vi "Main v0.01.vi"() -> ()   [LabVIEW 2017]
doc: "This vi is the main vi for startup. It has the following loops:\n\n1. The Event Handling Loop generates messages based on user interface actions.\n\n2. The Message Handling Loop processes messages generated by the Event Handling Loop, or by other messages. The messages are string values, so new messages can be added easily to the Message Cases case structure in the Message Handling Loop. Each message cluster can also provide an optional value for Message Data, which is a variant that can be converted to whatever message-specific data is required.\n\n3. The Auto Loop runs the endurance tests\n\n4. The Towerlight loop maintains the status of the towerlight based on machine running\n\n--------------------\n\nv1.7:\n- Added Sense ON Delay to the Tolerances Cluster making it user editable\n- Config file for writing tolerances is now changed to config.ini inside data folder\n\nv1.6:\n- Added a error dialog before starting loops to display errors\n- Backup nce file creation\n- UAC logger Updated\n\nv1.51:\n- Updated UAC\n\nChangelog\nv1.43:\n- Fixed bug for display of updated motor calibrration data (read new value from queue)\n- Fixed bug for speed calibration\n\nv1.41:\n- Added debouncing of E-Stop (Autoloop)\n- Modified timeout error algorithm (Procedure Run)\n- Text description on Settings screen\n\nv1.4:\n- Don;t allow to Run the test until correct procedure is selected\n\nv1.3:\n- UI updated for Calibration Screen\n\nv1.2:\n- UI Improvement:\n - Settings mode style updated\n\nv1.12:\n- Manual mode updated for ECU\n- Maintenance mode E-Stop colour changed\n\nv1.11:\n- Made towerlight handling into subVI\n\nv1.1:\n- Climate Chamber error convert to warning\n- View procedure puts same value into its indicators for next run. This basically means current procedure of the motor will show even if you do not change to another motor and return.\n- Added View Log feature\n- Added View Details feature\n\nv1.0:\n- Climate chamber integration completion\n- Maintenance mode along with climate UI\n- UI changes to auto screen\n\nv0.91:\n- Towerlight Buzzer intermittently\n- Remarks indicator added to Auto Mode\n\nv0.8:\n- Pause, Start, Stop, Procedure View updated\n- Diection indicator added\n- Motor Select enable/disable added\n\nv0.7:\n- Indicators & graphs updated for auto mode"
uses:
  support/Message Queue/Message Queue.lvlib
  <vilib>/Utility/error.llb/Error Cluster From Error Code.vi
  support/User Event - Stop/User Event - Stop.lvlib
  support/Message Queue/Enqueue Message (Single).vi
  <vilib>/ErrorRing/Error Ring.xnode
  support/GV/Towerlight GV.vi
  controls/Towerlight.ctl
  controls/FGV DO.ctl
  <resource>/objmgr/daqmx.rc
  controls/Auto States v0.2.ctl
  controls/AC Results.ctl
  controls/Update Measurements.ctl
  controls/Specifications.ctl
  controls/All Specs.ctl
  controls/Main Tabs.ctl
  controls/FGV AO.ctl
  GV/All Inputs.vi
  GV/Specs.vi
  controls/Model Name.ctl
  controls/Auto.ctl
  controls/SACB DI.ctl
panel:
  in  "Number":string="ID" caption="No"
  in  "Shift":string="ID"
  in  "BSL":bool
  out "Numeric Control":i32
  out "Array":string[](array[string])
  out "Total Time":dbl caption="Total Time (s)"
  in  "output cluster":T1={"LH"={"Go Up"={"Min Speed"=10.0, "Max Speed"=250.0, "Min Time"=0.5, "Max Time"=5.3, "Min Run Current"=0.0, "Max Run Current"=10.0, "Min Stall Current"=0.0, "Max Stall Current"=25.0, "Min Stall Force"=170.0, "Max Stall Force"=320.0, "Min Stroke"=170.0, "Max Stroke"=350.0}, "Go Down"={"Min Speed"=10.0, "Max Speed"=250.0, "Min Travel Time"=0.5, "Max Travel Time"=5.3, "Min Run Current"=0.0, "Max Run Current"=10.0}, "Shipping"={"Min Distance"=0.0, "Max Distance"=25.0, "Setpoint"=5.0}, "Anti-Pinch"={"Min Force"=5.0, "Max Force"=15.0}}, "RH"={"Go Up"={"Min Speed"=10.0, "Max Speed"=250.0, "Min Time"=0.5, "Max Time"=4.3, "Min Run Current"=0.0, "Max Run Current"=10.0, "Min Stall Current"=0.0, "Max Stall Current"=25.0, "Min Stall Force"=170.0, "Max Stall Force"=320.0, "Min Stroke"=170.0, "Max Stroke"=350.0}, "Go Down"={"Min Speed"=10.0, "Max Speed"=250.0, "Min Travel Time"=0.5, "Max Travel Time"=5.3, "Min Run Current"=0.0, "Max Run Current"=10.0}, "Shipping"={"Min Distance"=0.0, "Max Distance"=25.0, "Setpoint"=5.0}, "Anti-Pinch"={"Min Force"=5.0, "Max Force"=15.0}}, "W 601 FR RH Std"={"Go Up"={"Min Speed"=10.0, "Max Speed"=250.0, "Min Time"=0.5, "Max Time"=4.3, "Min Run Current"=0.0, "Max Run Current"=10.0, "Min Stall Current"=0.0, "Max Stall Current"=25.0, "Min Stall Force"=170.0, "Max Stall Force"=320.0, "Min Stroke"=254.4, "Max Stroke"=270.4}, "Go Down"={"Min Speed"=10.0, "Max Speed"=250.0, "Min Travel Time"=0.5, "Max Travel Time"=4.3, "Min Run Current"=0.0, "Max Run Current"=10.0}, "Shipping"={"Min Distance"=5.0, "Max Distance"=15.0, "Setpoint"=5.0}, "Anti-Pinch"={"Min Force"=5.0, "Max Force"=15.0}}, "W 601 FR LH Std"={"Go Up"={"Min Speed"=10.0, "Max Speed"=250.0, "Min Time"=0.5, "Max Time"=4.3, "Min Run Current"=0.0, "Max Run Current"=10.0, "Min Stall Current"=0.0, "Max Stall Current"=25.0, "Min Stall Force"=170.0, "Max Stall Force"=320.0, "Min Stroke"=254.4, "Max Stroke"=270.4}, "Go Down"={"Min Speed"=10.0, "Max Speed"=250.0, "Min Travel Time"=0.5, "Max Travel Time"=4.3, "Min Run Current"=0.0, "Max Run Current"=10.0}, "Shipping"={"Min Distance"=5.0, "Max Distance"=15.0, "Setpoint"=5.0}, "Anti-Pinch"={"Min Force"=5.0, "Max Force"=15.0}}, "W 601 RR RH Std"={"Go Up"={"Min Speed"=10.0, "Max Speed"=250.0, "Min Time"=0.5, "Max Time"=4.3, "Min Run Current"=0.0, "Max Run Current"=10.0, "Min Stall Current"=0.0, "Max Stall Current"=25.0, "Min Stall Force"=170.0, "Max Stall Force"=320.0, "Min Stroke"=254.4, "Max Stroke"=270.4}, "Go Down"={"Min Speed"=10.0, "Max Speed"=250.0, "Min Travel Time"=0.5, "Max Travel Time"=4.3, "Min Run Current"=0.0, "Max Run Current"=10.0}, "Shipping"={"Min Distance"=5.0, "Max Distance"=15.0, "Setpoint"=5.0}, "Anti-Pinch"={"Min Force"=5.0, "Max Force"=15.0}}, "W 601 RR LH Std"={"Go Up"={"Min Speed"=10.0, "Max Speed"=250.0, "Min Time"=0.5, "Max Time"=4.3, "Min Run Current"=0.0, "Max Run Current"=10.0, "Min Stall Current"=0.0, "Max Stall Current"=25.0, "Min Stall Force"=170.0, "Max Stall Force"=320.0, "Min Stroke"=254.4, "Max Stroke"=270.4}, "Go Down"={"Min Speed"=10.0, "Max Speed"=250.0, "Min Travel Time"=0.5, "Max Travel Time"=4.3, "Min Run Current"=0.0, "Max Run Current"=10.0}, "Shipping"={"Min Distance"=5.0, "Max Distance"=15.0, "Setpoint"=5.0}, "Anti-Pinch"={"Min Force"=5.0, "Max Force"=15.0}}, "W 601 FR RH AP"={"Go Up"={"Min Speed"=10.0, "Max Speed"=250.0, "Min Time"=0.5, "Max Time"=4.3, "Min Run Current"=0.0, "Max Run Current"=10.0, "Min Stall Current"=0.0, "Max Stall Current"=25.0, "Min Stall Force"=170.0, "Max Stall Force"=320.0, "Min Stroke"=254.4, "Max Stroke"=270.4}, "Go Down"={"Min Speed"=10.0, "Max Speed"=250.0, "Min Travel Time"=0.5, "Max Travel Time"=4.3, "Min Run Current"=0.0, "Max Run Current"=10.0}, "Shipping"={"Min Distance"=5.0, "Max Distance"=15.0, "Setpoint"=5.0}, "Anti-Pinch"={"Min Force"=5.0, "Max Force"=15.0}}, "W 601 FR LH AP"={"Go Up"={"Min Speed"=10.0, "Max Speed"=250.0, "Min Time"=0.5, "Max Time"=4.3, "Min Run Current"=0.0, "Max Run Current"=10.0, "Min Stall Current"=0.0, "Max Stall Current"=25.0, "Min Stall Force"=170.0, "Max Stall Force"=320.0, "Min Stroke"=254.4, "Max Stroke"=270.4}, "Go Down"={"Min Speed"=10.0, "Max Speed"=250.0, "Min Travel Time"=0.5, "Max Travel Time"=4.3, "Min Run Current"=0.0, "Max Run Current"=10.0}, "Shipping"={"Min Distance"=5.0, "Max Distance"=15.0, "Setpoint"=5.0}, "Anti-Pinch"={"Min Force"=5.0, "Max Force"=15.0}}, "W 601 RR RH AP"={"Go Up"={"Min Speed"=10.0, "Max Speed"=250.0, "Min Time"=0.5, "Max Time"=4.3, "Min Run Current"=0.0, "Max Run Current"=10.0, "Min Stall Current"=0.0, "Max Stall Current"=25.0, "Min Stall Force"=170.0, "Max Stall Force"=320.0, "Min Stroke"=254.4, "Max Stroke"=270.4}, "Go Down"={"Min Speed"=10.0, "Max Speed"=250.0, "Min Travel Time"=0.5, "Max Travel Time"=4.3, "Min Run Current"=0.0, "Max Run Current"=10.0}, "Shipping"={"Min Distance"=5.0, "Max Distance"=15.0, "Setpoint"=5.0}, "Anti-Pinch"={"Min Force"=5.0, "Max Force"=15.0}}, "W 601 RR LH AP"={"Go Up"={"Min Speed"=10.0, "Max Speed"=250.0, "Min Time"=0.5, "Max Time"=4.3, "Min Run Current"=0.0, "Max Run Current"=10.0, "Min Stall Current"=0.0, "Max Stall Current"=25.0, "Min Stall Force"=170.0, "Max Stall Force"=320.0, "Min Stroke"=254.4, "Max Stroke"=270.4}, "Go Down"={"Min Speed"=10.0, "Max Speed"=250.0, "Min Travel Time"=0.5, "Max Travel Time"=4.3, "Min Run Current"=0.0, "Max Run Current"=10.0}, "Shipping"={"Min Distance"=5.0, "Max Distance"=15.0, "Setpoint"=5.0}, "Anti-Pinch"={"Min Force"=5.0, "Max Force"=15.0}}}
  in  "Keyboard 2":bool
  out "TS Status":cluster{"Status":string, "Elapsed Time":dbl}
  in  "Stall Force":bool
  out "File Path Control":path
  out "String":string caption="XBA EOL Tester v0.01"
  out "EOL":T3 caption="Main Menu"
  in  "Calibration":bool
  in  "Manual":bool
  in  "Autocycle":T4
  in  "Maintenance":bool
  in  "Settings":bool
  out "Testing Time (s)":dbl caption="Cycle Time"
  out "Set Voltage":dbl=12.5
  out "AC Graph":cluster{"Graph":dbl[], "Graph":dbl[]}(graph)
  out "Results":T5 {"Go Up"."Stall Force" format="%#.1f"; "Go Up"."Speed" format="%#.1f"; "Go Up"."Running Current" format="%#.2f"; "Go Up"."Up Stroke" format="%#.1f"; "Go Up"."Stall Current" format="%#.2f"; "Go Down"."Speed" format="%#.1f"; "Go Down"."Travel Time" format="%#.2f"; "Go Down"."Running Current" format="%#.2f"; "Shipping Position"."Shipping Position" format="%#.1f"}
  out "Model Name 2":string caption="Model Name"
  out "AC Pictures":u16(ring)
  in  "View Log":bool
  out "Counts":T6
  in  "Home Autocycle":bool
  out "Status":string
  in  "Stroke Sensor":cluster{"Slope":dbl, "Intercept":dbl}={"Slope"=10.0, "Intercept"=0.0} {"Intercept" format="%#.4f"; "Slope" format="%#.4f"}
  in  "Save":bool
  in  "Current":cluster{"Slope":dbl, "Intercept":dbl}={"Slope"=10.0, "Intercept"=0.0} caption="Current Sensor" {"Intercept" format="%#.4f"; "Slope" format="%#.4f"}
  in  "Load Cell":cluster{"Slope":dbl, "Intercept":dbl}={"Slope"=10.0, "Intercept"=0.0} {"Intercept" format="%#.4f"; "Slope" format="%#.4f"}
  in  "Home Calib":bool
  out "Shipping":cluster{"Shipping Position":dbl}
  in  "Shipping":dbl=200.0 caption="Stop Motor for Shipping Position"
  out "manual error":errorcluster
  out "GO UP":T7
  out "GO DOWN":T8
  in  "Load?":bool caption="With\nLoad?"
  in  "Shipping Position":bool
  in  "Go Down":bool
  in  "Go Up":bool
  in  "Homing":bool
  out "Manual Graph":dbl[][](graph)
  in  "De-Clamp":bool
  out "StatusManual":cluster{"Status":string, "Elapsed Time":dbl}
  in  "Model Name":T9
  in  "Clamp":bool
  in  "Home Manual":bool
  in  "Settings Mode Change":T10(ring)
  in  "Print":bool
  in  "ID":string="ID"
  in  "Part Name":string="FRONT ELECTRIC WR - W501"
  in  "Part Number":string="23585284"
  in  "Settings Tab Control":T11(tab)
  in  "LH":T2={"Go Up"={"Min Speed"=20.0, "Max Speed"=200.0, "Min Time"=1.0, "Max Time"=4.3, "Min Run Current"=0.0, "Max Run Current"=10.0, "Min Stall Current"=0.0, "Max Stall Current"=25.0, "Min Stall Force"=170.0, "Max Stall Force"=320.0, "Min Stroke"=259.4, "Max Stroke"=264.4}, "Go Down"={"Min Speed"=20.0, "Max Speed"=200.0, "Min Travel Time"=1.0, "Max Travel Time"=4.3, "Min Run Current"=0.0, "Max Run Current"=10.0}, "Shipping"={"Min Distance"=5.0, "Max Distance"=15.0, "Setpoint"=5.0}, "Anti-Pinch"={"Min Force"=5.0, "Max Force"=15.0}}
  in  "RH":T2={"Go Up"={"Min Speed"=20.0, "Max Speed"=200.0, "Min Time"=1.0, "Max Time"=4.3, "Min Run Current"=0.0, "Max Run Current"=10.0, "Min Stall Current"=0.0, "Max Stall Current"=25.0, "Min Stall Force"=170.0, "Max Stall Force"=320.0, "Min Stroke"=259.4, "Max Stroke"=264.4}, "Go Down"={"Min Speed"=20.0, "Max Speed"=200.0, "Min Travel Time"=1.0, "Max Travel Time"=4.3, "Min Run Current"=0.0, "Max Run Current"=10.0}, "Shipping"={"Min Distance"=5.0, "Max Distance"=15.0, "Setpoint"=5.0}, "Anti-Pinch"={"Min Force"=5.0, "Max Force"=15.0}}
  in  "W 601 FR RH Std":T2={"Go Up"={"Min Speed"=20.0, "Max Speed"=200.0, "Min Time"=1.0, "Max Time"=4.3, "Min Run Current"=0.0, "Max Run Current"=10.0, "Min Stall Current"=0.0, "Max Stall Current"=25.0, "Min Stall Force"=170.0, "Max Stall Force"=320.0, "Min Stroke"=259.4, "Max Stroke"=264.4}, "Go Down"={"Min Speed"=20.0, "Max Speed"=200.0, "Min Travel Time"=1.0, "Max Travel Time"=4.3, "Min Run Current"=0.0, "Max Run Current"=10.0}, "Shipping"={"Min Distance"=5.0, "Max Distance"=15.0, "Setpoint"=5.0}, "Anti-Pinch"={"Min Force"=5.0, "Max Force"=15.0}}
  in  "W 601 FR LH Std":T2={"Go Up"={"Min Speed"=20.0, "Max Speed"=200.0, "Min Time"=1.0, "Max Time"=4.3, "Min Run Current"=0.0, "Max Run Current"=10.0, "Min Stall Current"=0.0, "Max Stall Current"=25.0, "Min Stall Force"=170.0, "Max Stall Force"=320.0, "Min Stroke"=259.4, "Max Stroke"=264.4}, "Go Down"={"Min Speed"=20.0, "Max Speed"=200.0, "Min Travel Time"=1.0, "Max Travel Time"=4.3, "Min Run Current"=0.0, "Max Run Current"=10.0}, "Shipping"={"Min Distance"=5.0, "Max Distance"=15.0, "Setpoint"=5.0}, "Anti-Pinch"={"Min Force"=5.0, "Max Force"=15.0}}
  in  "W 601 RR RH Std":T2={"Go Up"={"Min Speed"=20.0, "Max Speed"=200.0, "Min Time"=1.0, "Max Time"=4.3, "Min Run Current"=0.0, "Max Run Current"=10.0, "Min Stall Current"=0.0, "Max Stall Current"=25.0, "Min Stall Force"=170.0, "Max Stall Force"=320.0, "Min Stroke"=259.4, "Max Stroke"=264.4}, "Go Down"={"Min Speed"=20.0, "Max Speed"=200.0, "Min Travel Time"=1.0, "Max Travel Time"=4.3, "Min Run Current"=0.0, "Max Run Current"=10.0}, "Shipping"={"Min Distance"=5.0, "Max Distance"=15.0, "Setpoint"=5.0}, "Anti-Pinch"={"Min Force"=5.0, "Max Force"=15.0}}
  in  "W 601 RR LH Std":T2={"Go Up"={"Min Speed"=20.0, "Max Speed"=200.0, "Min Time"=1.0, "Max Time"=4.3, "Min Run Current"=0.0, "Max Run Current"=10.0, "Min Stall Current"=0.0, "Max Stall Current"=25.0, "Min Stall Force"=170.0, "Max Stall Force"=320.0, "Min Stroke"=259.4, "Max Stroke"=264.4}, "Go Down"={"Min Speed"=20.0, "Max Speed"=200.0, "Min Travel Time"=1.0, "Max Travel Time"=4.3, "Min Run Current"=0.0, "Max Run Current"=10.0}, "Shipping"={"Min Distance"=5.0, "Max Distance"=15.0, "Setpoint"=5.0}, "Anti-Pinch"={"Min Force"=5.0, "Max Force"=15.0}}
  in  "W 601 FR RH AP":T2={"Go Up"={"Min Speed"=20.0, "Max Speed"=200.0, "Min Time"=1.0, "Max Time"=4.3, "Min Run Current"=0.0, "Max Run Current"=10.0, "Min Stall Current"=0.0, "Max Stall Current"=25.0, "Min Stall Force"=170.0, "Max Stall Force"=320.0, "Min Stroke"=259.4, "Max Stroke"=264.4}, "Go Down"={"Min Speed"=20.0, "Max Speed"=200.0, "Min Travel Time"=1.0, "Max Travel Time"=4.3, "Min Run Current"=0.0, "Max Run Current"=10.0}, "Shipping"={"Min Distance"=5.0, "Max Distance"=15.0, "Setpoint"=5.0}, "Anti-Pinch"={"Min Force"=5.0, "Max Force"=15.0}}
  in  "W 601 FR LH AP":T2={"Go Up"={"Min Speed"=20.0, "Max Speed"=200.0, "Min Time"=1.0, "Max Time"=4.3, "Min Run Current"=0.0, "Max Run Current"=10.0, "Min Stall Current"=0.0, "Max Stall Current"=25.0, "Min Stall Force"=170.0, "Max Stall Force"=320.0, "Min Stroke"=259.4, "Max Stroke"=264.4}, "Go Down"={"Min Speed"=20.0, "Max Speed"=200.0, "Min Travel Time"=1.0, "Max Travel Time"=4.3, "Min Run Current"=0.0, "Max Run Current"=10.0}, "Shipping"={"Min Distance"=5.0, "Max Distance"=15.0, "Setpoint"=5.0}, "Anti-Pinch"={"Min Force"=5.0, "Max Force"=15.0}}
  in  "W 601 RR RH AP":T2={"Go Up"={"Min Speed"=20.0, "Max Speed"=200.0, "Min Time"=1.0, "Max Time"=4.3, "Min Run Current"=0.0, "Max Run Current"=10.0, "Min Stall Current"=0.0, "Max Stall Current"=25.0, "Min Stall Force"=170.0, "Max Stall Force"=320.0, "Min Stroke"=259.4, "Max Stroke"=264.4}, "Go Down"={"Min Speed"=20.0, "Max Speed"=200.0, "Min Travel Time"=1.0, "Max Travel Time"=4.3, "Min Run Current"=0.0, "Max Run Current"=10.0}, "Shipping"={"Min Distance"=5.0, "Max Distance"=15.0, "Setpoint"=5.0}, "Anti-Pinch"={"Min Force"=5.0, "Max Force"=15.0}}
  in  "W 601 RR LH AP":T2={"Go Up"={"Min Speed"=20.0, "Max Speed"=200.0, "Min Time"=1.0, "Max Time"=4.3, "Min Run Current"=0.0, "Max Run Current"=10.0, "Min Stall Current"=0.0, "Max Stall Current"=25.0, "Min Stall Force"=170.0, "Max Stall Force"=320.0, "Min Stroke"=259.4, "Max Stroke"=264.4}, "Go Down"={"Min Speed"=20.0, "Max Speed"=200.0, "Min Travel Time"=1.0, "Max Travel Time"=4.3, "Min Run Current"=0.0, "Max Run Current"=10.0}, "Shipping"={"Min Distance"=5.0, "Max Distance"=15.0, "Setpoint"=5.0}, "Anti-Pinch"={"Min Force"=5.0, "Max Force"=15.0}}
  in  "Save Specs":bool
  in  "Home Settings":bool
  out "Reject Door SW":bool caption="Reject Sensor 2"
  in  "TareStroke":bool caption="Reset"
  in  "Pause":bool
  out "RS Loadcell Rear":bool
  out "RS Loadcell Front":bool
  in  "Loadcell CYL":bool caption="Load Cell CYL Front"
  out "RS Load UP Rear":bool
  out "RS Load UP Front":bool
  out "RS Load DN Rear":bool
  out "RS Load DN Front":bool
  in  "Load Lift Up Front":bool
  in  "Load Lift Up Rear":bool
  in  "Load Lift Dn Front":bool
  in  "Load Lift Dn Rear":bool
  in  "Average":bool caption="Filter ON?"
  in  "Reset Graph":bool caption="Reset"
  in  "Motor Short":bool
  in  "Clamp":bool
  in  "Home Maint":bool
  in  "Motor CW":bool
  in  "Motor CCW":bool
  out "Safety Curtain":bool
  out "Pressure":bool
  out "Machine ON":bool
  out "Start":bool
  out "Reject Sensor 1":bool
  out "Reject Sensor 2":bool
  out "E-Stop":bool
  in  "TL Red":bool caption="Towerlight Red"
  in  "TL Orange":bool caption="Towerlight Orange"
  in  "TL Green":bool caption="Towerlight Green"
  in  "TL Buzzer":bool caption="Towerlight Buzzer"
  in  "Motor ON":bool
  out "Current (A)":dbl
  out "Graph":dbl[][](graph)
  out "Load Cell (N)":dbl
  out "Stroke (mm)":dbl
  out "Connected?":bool
  out "SACB Inputs":T12
  in  "Exit":bool
  # "AAP WR EOL Testing Machine"
  # "Calibration Mode"
  # "Calibration mode allows you to change the calibration of (a)Analog Outputs such as Brake Load, and (b)Analog Inputs such as Torque, Current, Supply Voltage & Terminal Voltage."
  # "Calibration mode allows you to change the calibration of (a)Analog Outputs such as Brake Load, and (b)Analog Inputs such as Torque, Current, Supply Voltage & Terminal Voltage."
  # "RS_Clamping_top_Front\nRS_Clamping_bottom_Front\nRS_Clamping_MotorLH_Front\nRS_Clamping_MotorRH_Front\nIPS_Part presence_top_LH\nIPS_Part presence_Bottom_LH\nIPS_Part presence_top_RH\nIPS_Part presence_Bottom_RH\nIPS_Load engaged_1\nIPS_Part presence_2\nIPS_Load engaged_MCO_LH\nIPS_Load engaged_MCO_RH"
  # "Calibrate Torque, Current, & Voltage measurements are features that allow you to enter in measured values v/s expected values. The software will then automatically calculate and record each corresponding value into a table.\n\nFor example, in the graph shown on the right (fig.1), the actual raw analog input voltage is shown in the X-axis while the scaled value is shown in the Y-axis as \"Nm\" units."
  # "Calibrate Torque, Current, & Voltage measurements are features that allow you to enter in measured values v/s expected values. The software will then automatically calculate and record each corresponding value into a table.\n\nFor example, in the graph shown on the right (fig.1), the actual raw analog input voltage is shown in the X-axis while the scaled value is shown in the Y-axis as \"Nm\" units."
  # "Self-Calibrate Brake Magnet is an \"Auto-Calibration\" feature whereby the software will automatically record corresponding values of output voltage v/s torque measurement. It is recommended that you run this AFTER calibrating the torque sensor."
  # "Self-Calibrate Brake Magnet is an \"Auto-Calibration\" feature whereby the software will automatically record corresponding values of output voltage v/s torque measurement. It is recommended that you run this AFTER calibrating the torque sensor."
  # "2019 - Sasyaka Engineering Solutions, India - www.sasyaka.com"
  # "Calibration of Sensors"
  # "Details of Calibration"
  # "There are two types of sensors used in this machine: load cell and Current sensor.\t\t\t\t\t\n\t\t\t\t\t\nThe calibration data that can be entered here is the slope (M) and intercept (C). The scaled value (Y) is calculated as:\t\t\t\t\t\n\t\t\t\t\t\n                               Y = M*x + C\t\t\t\t\t\n                 Where 'x' is the raw electrical value.\t\t\t\t\t\n\t\t\t\t\t\nFor example, in the graph shown on the right (fig.1), the actual raw analog input voltage is shown in the X-axis while the scaled value is shown in the Y-axis as \"Nm\" units.\n\nPlease enter the appropriate values of m & c as per your calibration records."
  # "fig.1: Plot of Input Voltage v/s Torque"
  # "Results"
  # "Manual Mode"
  # "Settings & Parameters"
  # "Check Printer"
  # "You can test the printing facility here. (No changes can be made to actual text)"
  # "Sample Label shown above"
  # "Enter data for representative purposes and choose \"Test Print\" to print."
  # "Towerlight"
  # "Clamping CYL"
  # "Motor Control"
  # "Load Lifting CYL"
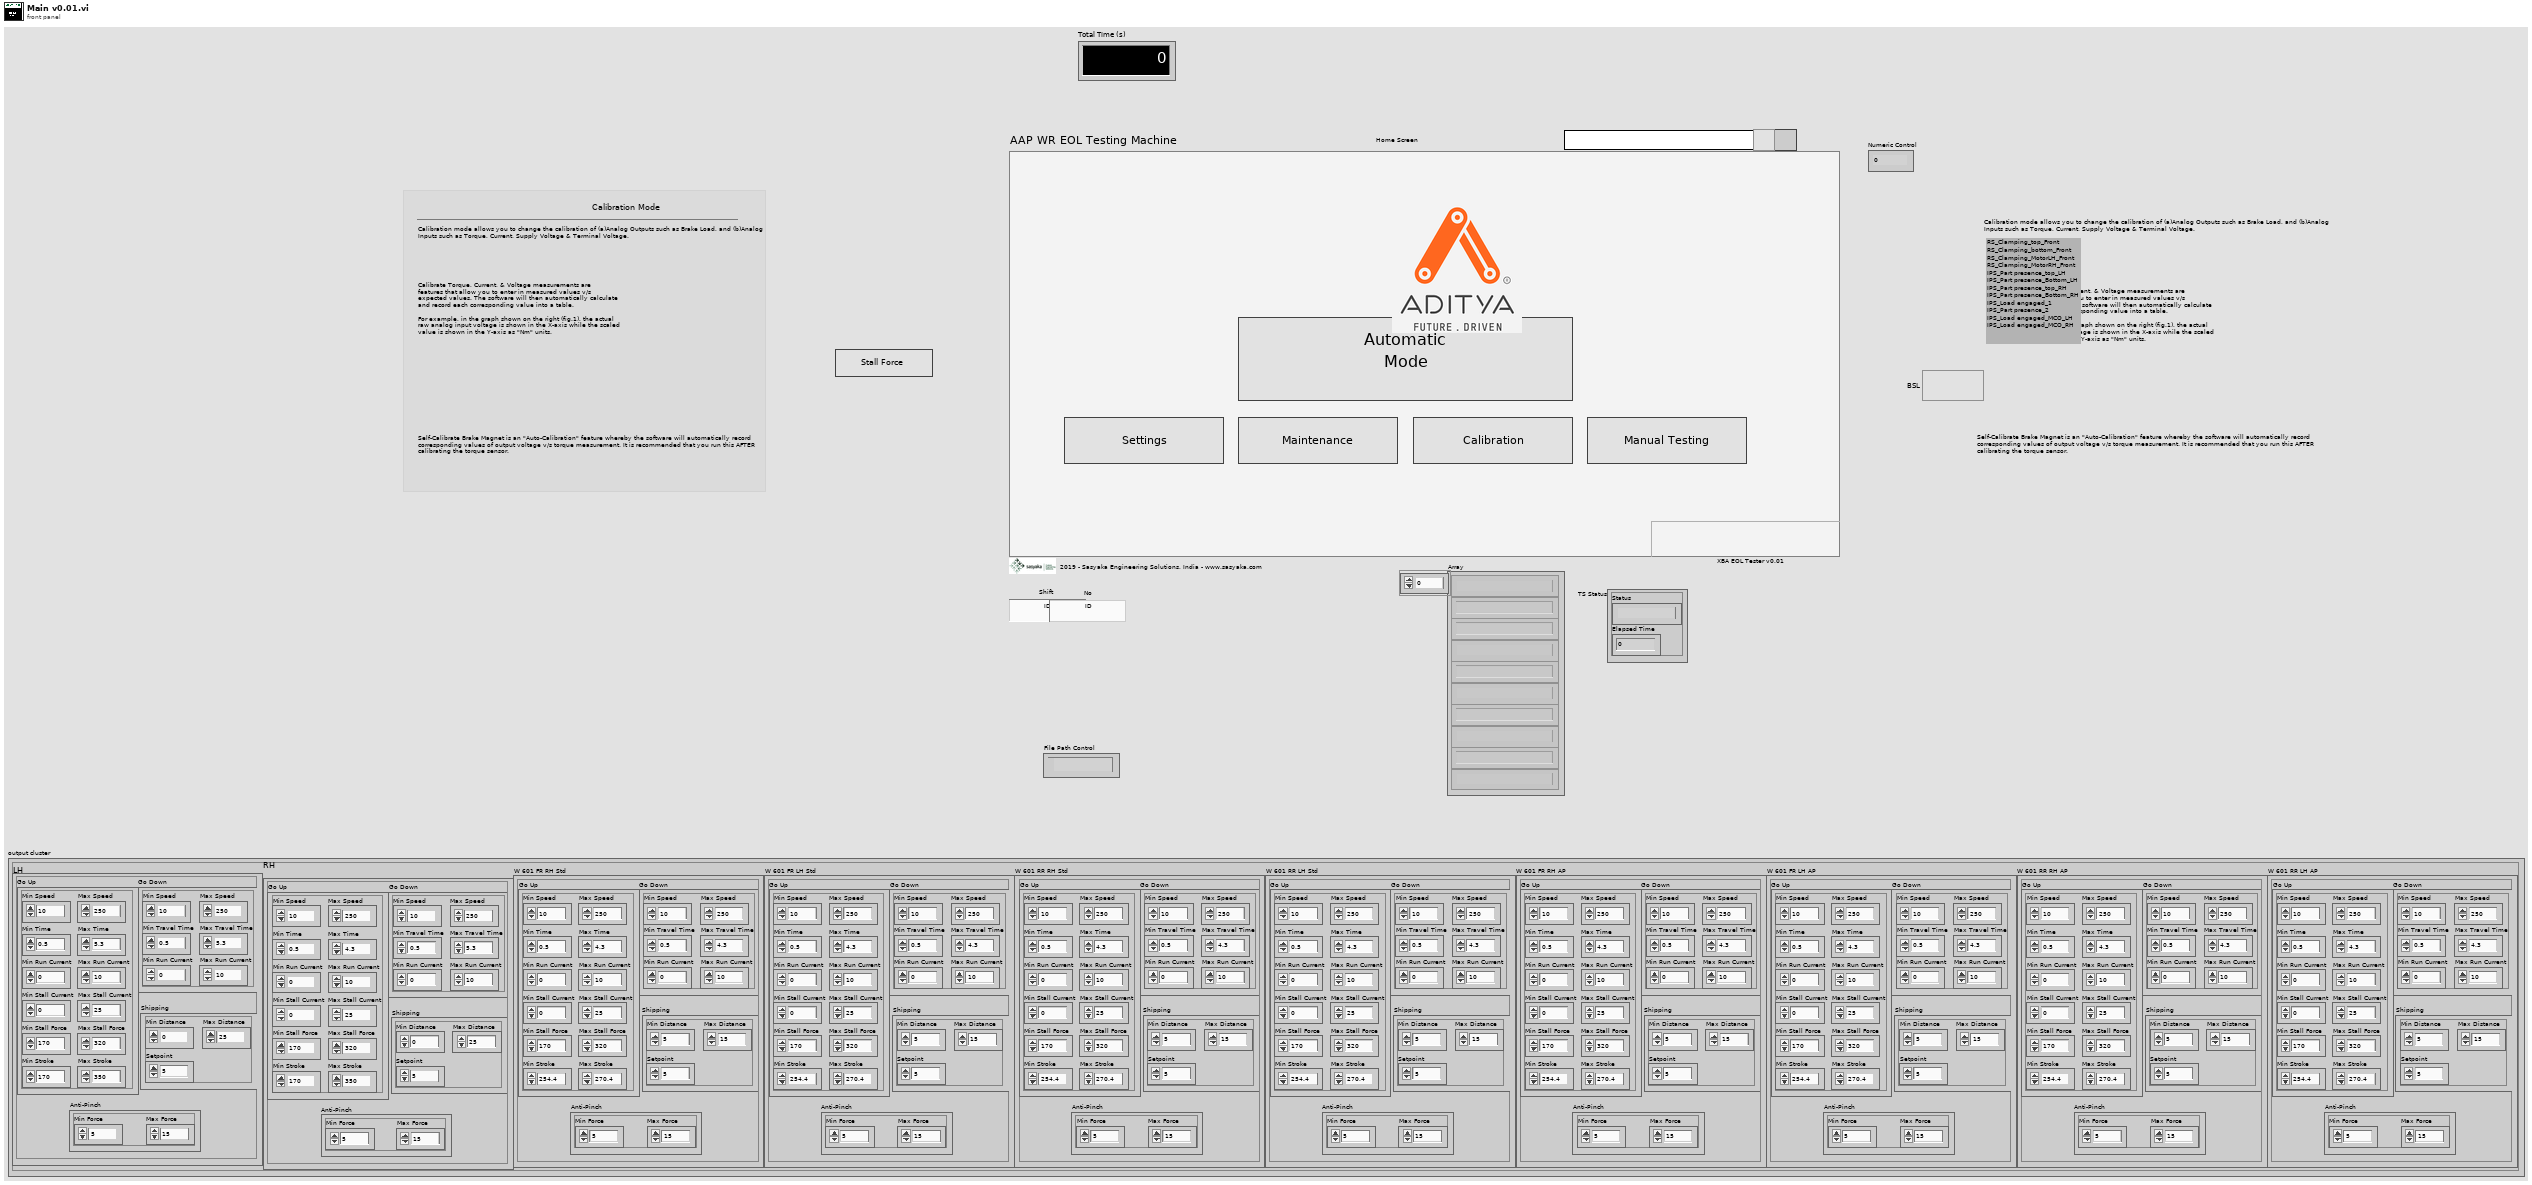
[diagram p1: front panel]
types:
  T1 = typedef "All Specs.ctl" = cluster{"LH":T2, "RH":T2, "W 601 FR RH Std":T2, "W 601 FR LH Std":T2, "W 601 RR RH Std":T2, "W 601 RR LH Std":T2, "W 601 FR RH AP":T2, "W 601 FR LH AP":T2, "W 601 RR RH AP":T2, "W 601 RR LH AP":T2}
  T2 = typedef "Specifications.ctl" = cluster{"Go Up":cluster{"Min Speed":dbl, "Max Speed":dbl, "Min Time":dbl, "Max Time":dbl, "Min Run Current":dbl, "Max Run Current":dbl, "Min Stall Current":dbl, "Max Stall Current":dbl, "Min Stall Force":dbl, "Max Stall Force":dbl, "Min Stroke":dbl, "Max Stroke":dbl}, "Go Down":cluster{"Min Speed":dbl, "Max Speed":dbl, "Min Travel Time":dbl, "Max Travel Time":dbl, "Min Run Current":dbl, "Max Run Current":dbl}, "Shipping":cluster{"Min Distance":dbl, "Max Distance":dbl, "Setpoint":dbl}, "Anti-Pinch":cluster{"Min Force":dbl, "Max Force":dbl}}
  T3 = typedef "Main Tabs.ctl" = enum32{"Home Screen", "Autocycle", "Calibration", "Manual Mode", "Settings", "Maintenance"}
  T4 = typedef "Auto.ctl" = bool
  T5 = typedef "AC Results.ctl" = cluster{"Initial":cluster{"Date":string, "Time":string, "ID":string}, "Go Up":cluster{"Speed":dbl, "Travel Time":dbl, "Running Current":dbl, "Up Stroke":dbl, "Stall Current":dbl, "Stall Force":dbl}, "Go Down":cluster{"Speed":dbl, "Travel Time":dbl, "Running Current":dbl, "Down Stroke":dbl}, "Shipping Position":cluster{"Shipping Position":dbl}, "Results":cluster{"PASS?":bool, "Details":string}}
  T6 = cluster{"TotalCount":u16, "PassCount":u16, "FailCount":u16}
  T7 = cluster{"Speed (mm/s)":dbl, "Travel Time (s)":dbl, "Run Current (A)":dbl, "Stroke":dbl, "Stall Current (A)":dbl, "Stall Force (N)":dbl}
  T8 = cluster{"Speed (mm/s)":dbl, "Travel Time (s)":dbl, "Running Current (A)":dbl, "Down Stroke":dbl}
  T9 = typedef "Model Name.ctl" = enum16{"W 501 FLH Std.", "W 501 FRH Std.", "W 601 FR RH Std", "W 601 FR LH Std", "W 601 RR RH Std", "W 601 RR LH Std", "W 601 FR RH AP", "W 601 FR LH AP", "W 601 RR RH AP", "W 601 RR LH AP"}
  T10 = enum16{"LH", "RH", "W 601 FR RH Std", "W 601 FR LH Std", "W 601 RR RH Std", "W 601 RR LH Std", "W 601 FR RH AP", "W 601 FR LH AP", "W 601 RR RH AP", "W 601 RR LH AP"}
  T11 = enum32{"LH", "RH", "W 601 FR RH Std", "W 601 FR LH Std", "W 601 RR RH Std", "W 601 RR LH Std", "W 601 FR RH AP", "W 601 FR LH AP", "W 601 RR RH AP", "W 601 RR LH AP"}
  T12 = typedef "SACB DI.ctl" = cluster{"RS ClampTop Front":bool, "RS ClampBottom Front":bool, "RS ClampMotorLH Front":bool, "RS ClampMotorRH Front":bool, "IPS PartPresenceTop LH":bool, "IPS PartPresenceBottom LH":bool, "IPS PartPresenceTop RH":bool, "IPS PartPresenceBottom RH":bool, "IPS LoadEngaged 1":bool, "IPS LoadEngaged 2":bool, "C10":bool, "C11":bool, "C12":bool, "C13":bool, "C14":bool, "C15":bool}
  T13 = typedef "FGV DO.ctl" = enum16{"Initialize", "Start Task", "Clamping", "Load CYL", "Contactors", "Loadcell CYL", "BSL", "Read DO", "Clear Tasks", "Clear Task"}
  T14 = enum32{"Invalid", "Standard", "Closed", "Hidden", "Minimized", "Maximized"}
  T15 = typedef "Semaphore RefNum" = refnum<k1>
  T16 = typedef "Message Queue.lvlib/All Message Queues.ctl" = cluster{"UI":refnum<queue>, "Auto":refnum<queue>}
  T17 = typedef "Towerlight.ctl" = enum16{"Idle", "Error", "Attention", "Running", "Maintenance", "Fail"}
  T18 = enum8{"Enabled", "Disabled", "Disabled and Grayed Out"}
  T19 = typedef "Auto States v0.2.ctl" = enum16{"Initialize", "Check Pressure", "Check EStop", "Check Reject Door ", "Check ReadyCondition", "Wait to Home", "Declamping", "Loadcell CYL to Home", "Wait for Part Presence", "Wait for Hands-Off", "Clamp", "Wait for Load Engage", "Wait for Start", "Test Sequencer", "Log & Print", "check for pass or fail", "Result", "Wait for Reject Door Open", "Wait for Reject 2 OFF", "Wait for Reject 2 ON", "Wait for Reject 1 OFF", "Wait for Reject 1 ON", "Wait for Reject Door Close"}
  T20 = typedef "Update Measurements.ctl" = cluster{"Results":T5, "TS Status":cluster{"Status":string, "Elapsed Time":dbl}, "Counts":cluster{"TotalCount":u16, "PassCount":u16, "FailCount":u16}, "AC Graph":cluster{"X":dbl, "Y":dbl}[], "Total Time":dbl, "Testing Time (s)":dbl, "Graph":dbl[][], "signal out":waveform(dbl)}
  T21 = typedef "FGV AO.ctl" = enum16{"Initialize", "Write AO", "Clear Tasks"}
  T22 = cluster{"Exit":refnum<vi>, "EOL":refnum<vi>, "Settings Tab Control":refnum<vi>}
  T23 = cluster{"task out":refnum<k21>, "task out":refnum<k21>, "task out":refnum<k21>}
  T24 = typedef "All Inputs.ctl" = cluster{"DI":cluster{"Machine ON":bool, "E-Stop":bool, "Pressure":bool, "Start":bool, "Safety Curtain":bool, "RS Load UP Rear":bool, "RS Load UP Front":bool, "RS Load DN Rear":bool, "RS Load DN Front":bool, "RS Loadcell Rear":bool, "RS Loadcell Front":bool, "Reject Sensor 1":bool, "Reject Sensor 2":bool, "Door SW Reject":bool}, "AI":cluster{"Force":dbl[], "Stroke":dbl[], "CurrentMon":dbl[]}, "SACB Inputs":T12}
  T25 = cluster{"Speed":dbl, "Travel Time":dbl, "Running Current":dbl, "Up Stroke":dbl, "Stall Current":dbl, "Stall Force":dbl}
  T26 = cluster{"Speed":dbl, "Travel Time":dbl, "Running Current":dbl, "Down Stroke":dbl}
  T27 = cluster{"Model Name":T9, "ID":string, "Shift":string}
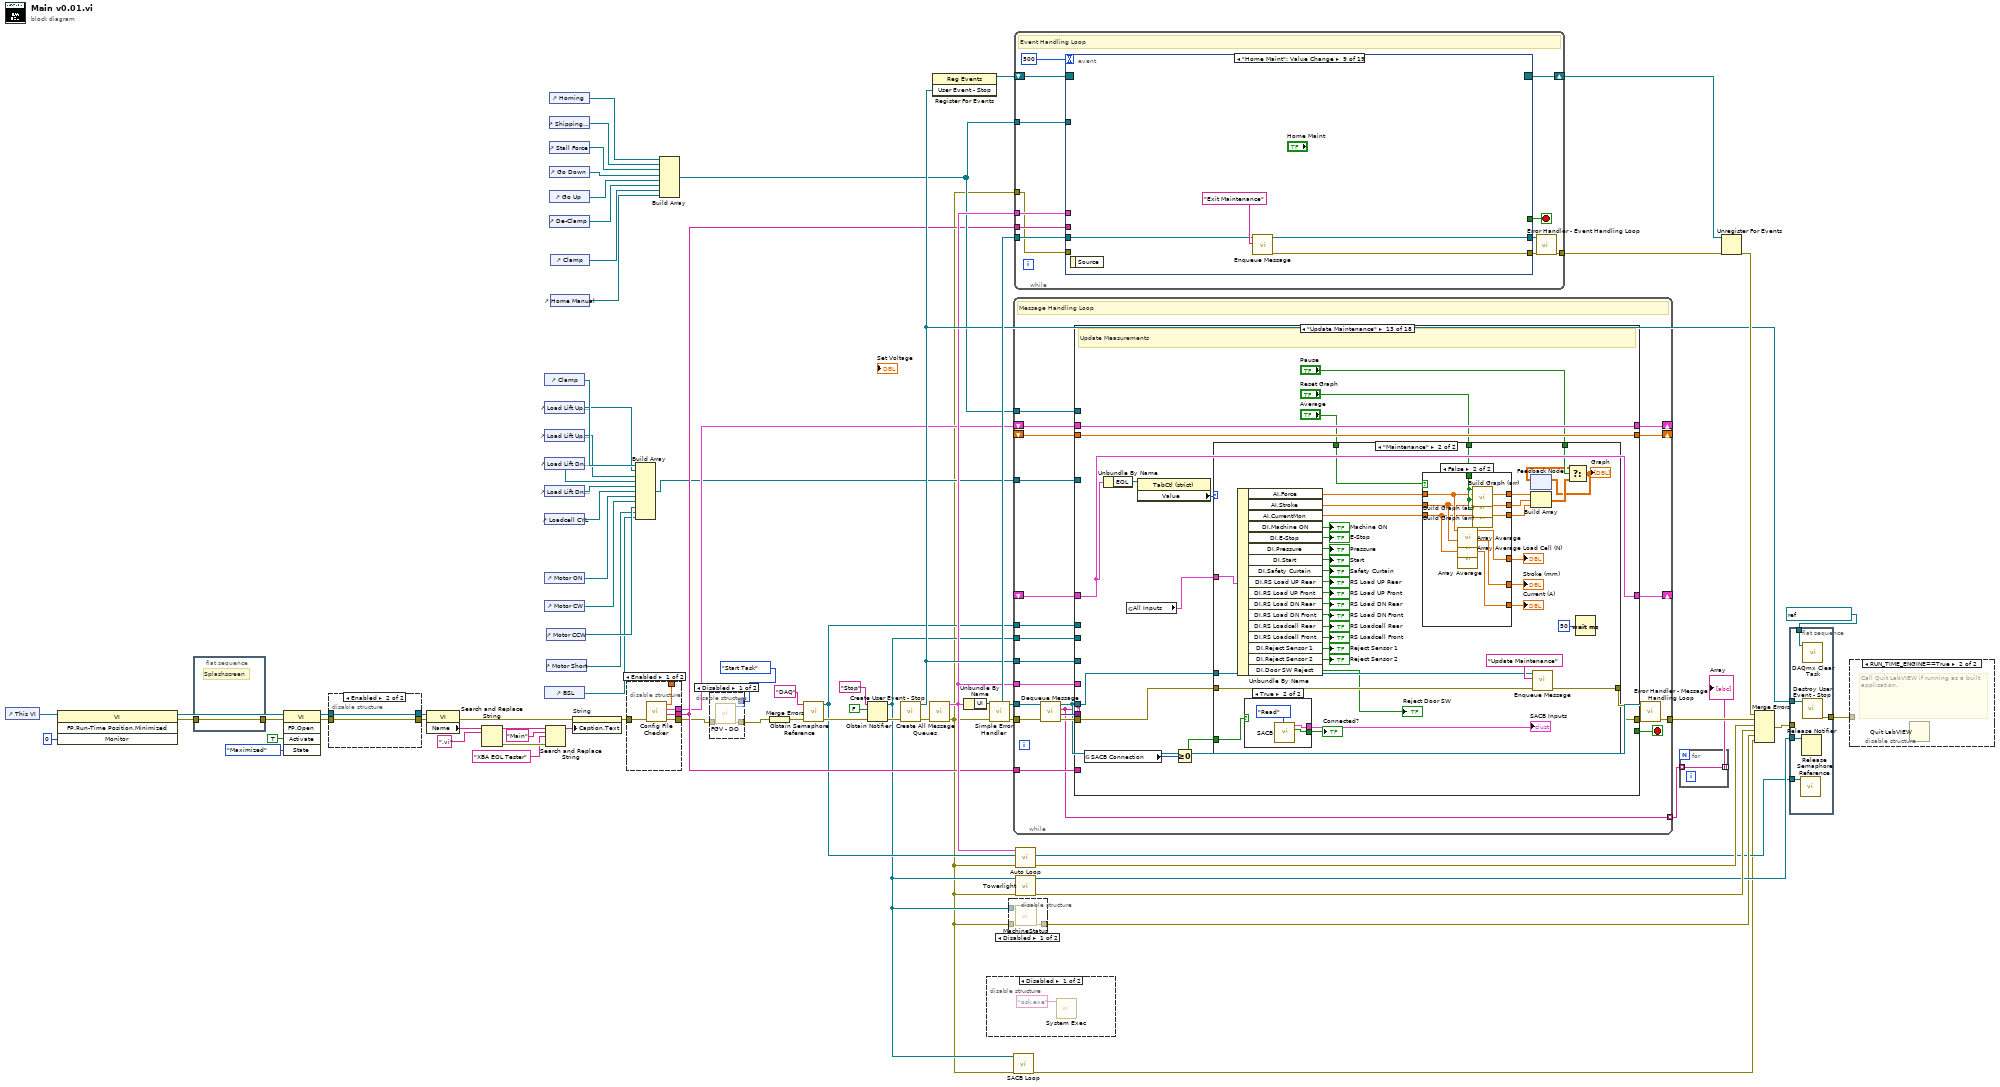
[diagram p0: block diagram]
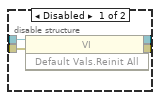
[diagram p4: hidden frame]
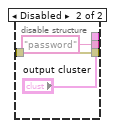
[diagram p5: hidden frame]
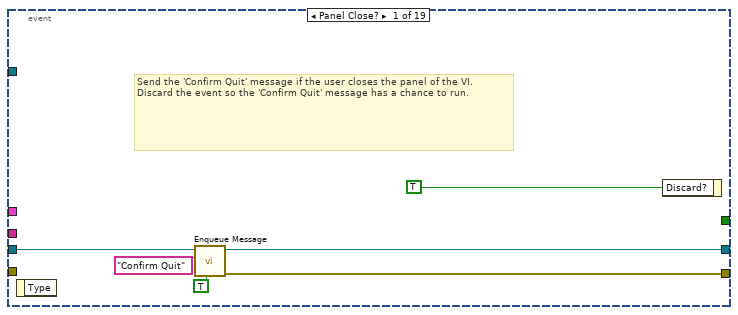
[diagram p7: hidden frame]
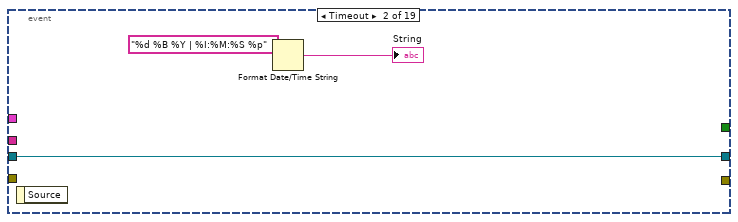
[diagram p8: hidden frame]
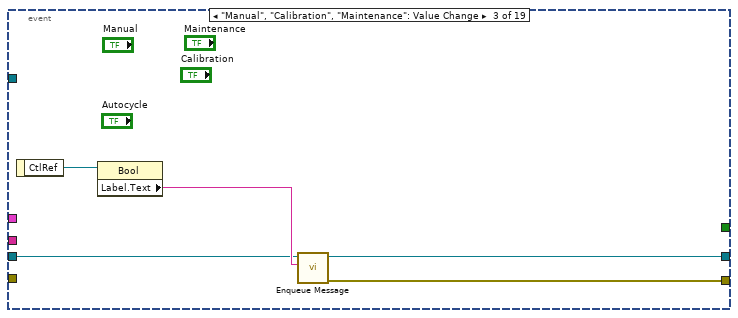
[diagram p9: hidden frame]
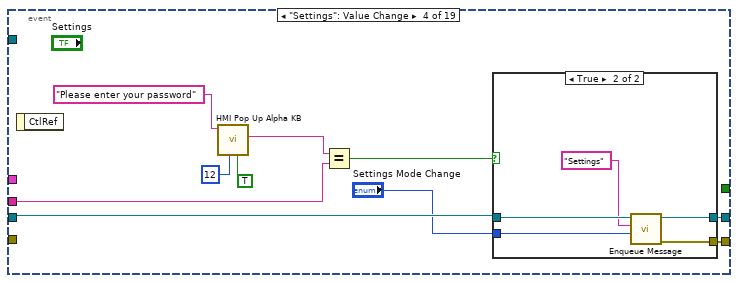
[diagram p10: hidden frame]
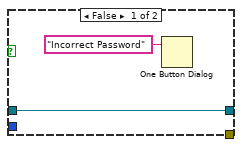
[diagram p11: hidden frame]
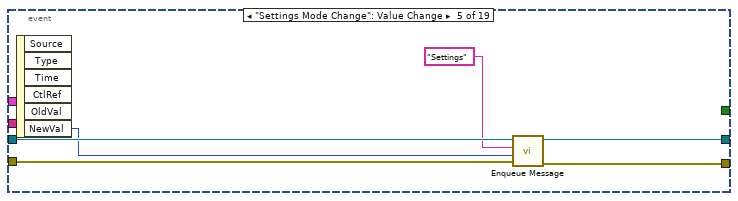
[diagram p12: hidden frame]
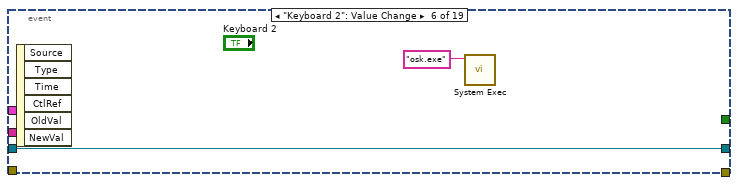
[diagram p13: hidden frame]
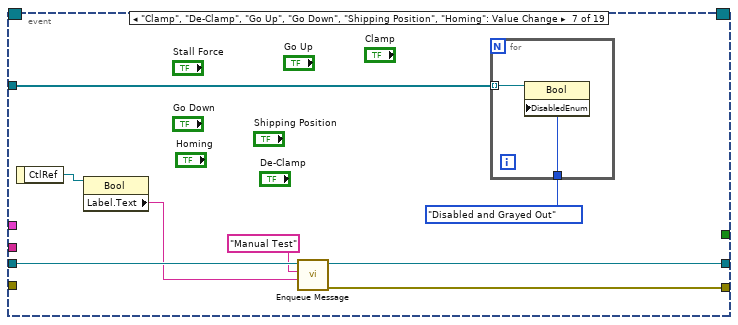
[diagram p14: hidden frame]
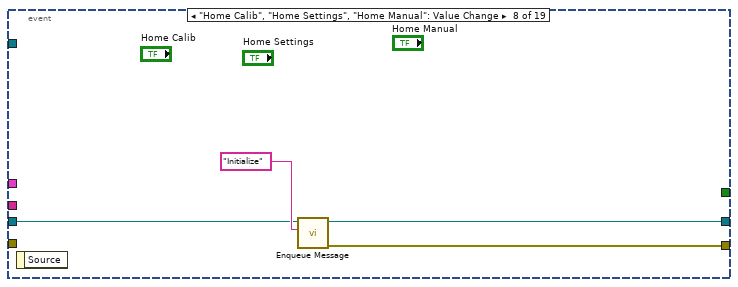
[diagram p15: hidden frame]
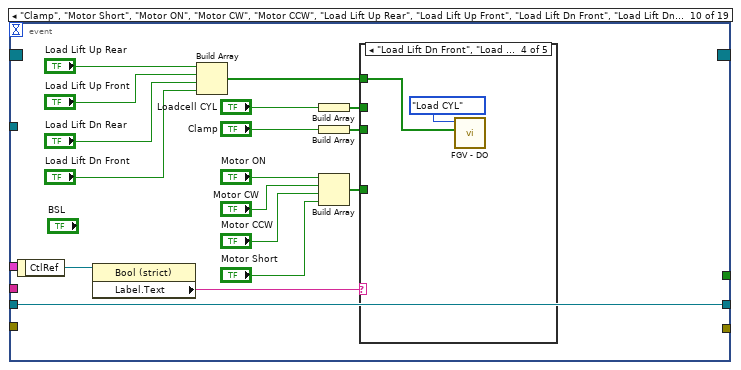
[diagram p16: hidden frame]
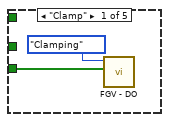
[diagram p17: hidden frame]
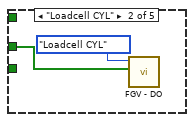
[diagram p18: hidden frame]
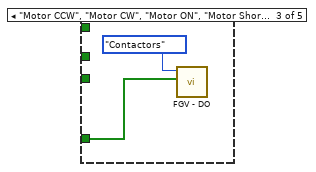
[diagram p19: hidden frame]
diagram:
  n1 = control-ref of="This VI"() -> (w58:refnum<vi>)
  n2 = invoke class="VI" method="FP.Run-Time Position.Minimized"(reference=w58, "Monitor"=i16 0) -> (reference out=w59:refnum<vi>, error out=w41:errorcluster)  [unwired: 2 in, 2 out]
  n3 = flat-sequence {
    tunnel: w41 -> [w77]
    tunnel: [w77] -> w40
    frame #0 {
      # "Splashscreen"
    }
  }
  n4 = invoke class="VI" method="FP.Open"(reference=w59, error in=w40, "Activate"=TRUE ("Activate?"), "State"=T14."Maximized") -> (reference out=w45:refnum<vi>, error out=w44:errorcluster)  [unwired: 1 in, 3 out]
  n5 = disable-structure shown="Enabled" {
    disable-tunnel: [w81 w83] -> w47
    disable-tunnel: [w80 w82] -> w46
    disable-tunnel: w45 -> [w79 w82]
    disable-tunnel: w44 -> [w78 w83]
    frame Disabled {
      n6 = invoke class="VI" method="Default Vals.Reinit All"(reference=w79, error in=w78) -> (reference out=w80:refnum<vi>, error out=w81:errorcluster)  [unwired: 1 in, 1 out]
    }
    frame Enabled {
    }
  }
  n7 = property class="VI"(reference=w46, error in=w47) -> (error out=w53:errorcluster, "Name"=w55:string)  [unwired: 1 out]
  n8 = Search and Replace String(input string=w55, search string=".vi") -> (result string=w52:string, error out=w51:errorcluster)  [unwired: 6 in, 2 out]
  n9 = control-ref of="Clamp"() -> (w15:refnum<vi>)
  n10 = control-ref of="Load Lift Up Front"() -> (w14:refnum<vi>)
  n11 = control-ref of="Load Lift Up Rear"() -> (w13:refnum<vi>)
  n12 = control-ref of="Load Lift Dn Front"() -> (w12:refnum<vi>)
  n13 = control-ref of="Load Lift Dn Rear"() -> (w11:refnum<vi>)
  n14 = control-ref of="Loadcell CYL"() -> (w10:refnum<vi>)
  n15 = control-ref of="Motor ON"() -> (w9:refnum<vi>)
  n16 = control-ref of="Motor CW"() -> (w8:refnum<vi>)
  n17 = control-ref of="BSL"() -> (w4:refnum<vi>)
  n18 = Search and Replace String(input string=w52, search string="Main", replace string="XBA EOL Tester" ("replace string (\"\")"), error in=w51) -> (result string=w48:string)  [unwired: 4 in, 3 out]
  n19 = control-ref of="Motor CCW"() -> (w6:refnum<vi>)
  n20 = control-ref of="Motor Short"() -> (w5:refnum<vi>)
  n21 = control-ref of="Homing"() -> (w22:refnum<vi>)
  n22 = control-ref of="Shipping Position"() -> (w23:refnum<vi>)
  n23 = control-ref of="Stall Force"() -> (w24:refnum<vi>)
  n24 = control-ref of="Go Down"() -> (w25:refnum<vi>)
  n25 = control-ref of="Go Up"() -> (w26:refnum<vi>)
  n26 = control-ref of="De-Clamp"() -> (w27:refnum<vi>)
  n27 = control-ref of="Clamp"() -> (w38:refnum<vi>)
  n28 = control-ref of="Home Manual"() -> (w37:refnum<vi>)
  n29 = property on="String" class="Str"(error in=w53, "Caption.Text"=w48) -> (error out=w35:errorcluster)  [unwired: 1 in, 1 out]
  n30 = disable-structure shown="Enabled" {
    disable-tunnel: w35 -> [w88 w91]
    disable-tunnel: [w87 "output cluster"] -> w21
    disable-tunnel: [w86 w91] -> w19
    disable-tunnel: [w85 "password" ("Password")] -> w34
    disable-tunnel: [w84 _] -> _
    frame Enabled {
      n31 = call "Config File Checker.vi"("Error In"=w88) -> ("error out"=w86:errorcluster, "Password"=w85:string, "output cluster"=w87:T1, "Shipping"=w84:dbl)  [unwired: 7 in]
    }
    frame Disabled {
    }
  }
  n32 = Build Array(w15, w14, w13, w12, w11, w10, w9, w8, w6, w5, w4) -> (w7:refnum<vi>[])
  n33 = Build Array(w22, w23, w24, w25, w26, w27, w38, w37) -> (w36:refnum<vi>[])
  n34 = disable-structure shown="Disabled" {
    disable-tunnel: FGV_DO."Start Task" ("State") -> [w94 _]
    disable-tunnel: w19 -> [w93 _]
    disable-tunnel: [w92 _] -> w18
    frame Disabled {
      n35 = call "FGV - DO.vi"("error in"=w93, "State"=w94) -> ("error out"=w92:errorcluster)  [unwired: 8 in, 1 out]
    }
    frame Enabled {
    }
  }
  n36 = Merge Errors(w18) -> (w32:errorcluster)
  n37 = call <vilib>:"Obtain Semaphore Reference.vi"("error in (no error)"=w32, "name (unnamed)"="DAQ") -> ("error out"=w31:errorcluster, "semaphore"=w28:T15)  [unwired: 3 in, 1 out]
  n38 = Obtain Notifier(name (unnamed)="Stop", notification data type=FALSE ("Stop Button"), error in (no error)=w31) -> (notifier out=w3:refnum<notifier>, error out=w63:errorcluster)  [unwired: 1 in, 1 out]
  n39 = call "Create User Event - Stop.vi"("error in (no error)"=w63) -> ("error out"=w74:errorcluster, "User Event - Stop"=w67:refnum<user-event>)  [unwired: 9 in]
  n40 = call "Create All Message Queues.vi"("error in (no error)"=w74) -> ("error out"=w2:errorcluster, "Message Queues out"=w64:T16)  [unwired: 9 in]
  n41 = register-events(w67) -> (reference out=w68:refnum<event-registration>)  [unwired: 2 in, 1 out]
  n42 = Unbundle By Name(w64) -> ("UI"=w75:refnum<queue>)
  n43 = disable-structure shown="Disabled" {
    frame Disabled {
      n44 = call <vilib>:"System Exec.vi"("command line"="osk.exe") -> ()  [unwired: 7 in, 4 out]
    }
    frame Enabled {
    }
  }
  n45 = call <vilib>:"Simple Error Handler.vi"("error in (no error)"=w2) -> ("error out"=w56:errorcluster)  [unwired: 4 in, 4 out]
  n46 = disable-structure shown="Disabled" {
    disable-tunnel: w3 -> [w98 _]
    disable-tunnel: [w97 _] -> w39
    disable-tunnel: w2 -> [w96 _]
    frame Disabled {
      n47 = call "MachineStatus.vi"("Error"=w96, "notifier in"=w98) -> ("outError"=w97:errorcluster)  [unwired: 9 in]
    }
    frame Enabled {
    }
  }
  n48 = call "SACB Loop.vi"("error in"=w2, "Notifier in"=w3) -> ("error out"=w1:errorcluster)  [unwired: 8 in, 1 out]
  n49 = while {
    tunnel: w75 -> [w113]
    shift-right: [w119] -> _
    shift-left: _ -> [w120]
    tunnel: w67 -> [w117]
    tunnel: w56 -> [w116]
    tunnel: [w112] -> w76
    tunnel: w64 -> [w110]
    shift-right: [w109] -> _
    shift-left: _ -> [w108]
    shift-right: [w107] -> _
    shift-left: w21 -> [w106]
    tunnel: w3 -> [w104]
    tunnel: w36 -> [w103]
    tunnel: w34 -> [w102]
    tunnel: w28 -> [w101]
    tunnel: [w100] -> w17 mode=indexing
    tunnel: w7 -> [w99]
    stop <- w118 stop-if-true
    # "Message Handling Loop"
    n50 = call "Dequeue Message.vi"("error in (no error)"=w116, "Message Queue"=w113) -> ("error out"=w115:errorcluster, "Message Data"=w114:variant, "Message"=w100:string, "dup Message Queue"=w105:refnum<queue>)  [unwired: 6 in]
    n51 = case "Message Cases" shown="\"Update Maintenance\"" w100 {
      selector: w100 -> [_ _ _ _ _ _ _ _ _ _ _ _ _ _ _ _ _ w606]
      tunnel: w105 -> [_ _ w144 _ w264 _ _ _ _ _ _ _ w477 w549 _ w570 w603 _]
      tunnel: w115 -> [w126 w135 w148 w177 w267 w277 w308 w339 w360 w375 w402 w470 w478 w551 w564 w574 w596 _]
      tunnel: [w125 w137 w142 w161 w265 w277 w298 w339 w354 w376 w401 w463 w476 w550 w558 w572 w599 w607] -> w111
      tunnel: w120 -> [_ w136 w149 w181 w269 w276 w316 w342 w365 w378 w403 w471 w482 w555 w563 w573 w602 w608]
      tunnel: [w131 w136 w149 w181 w269 w276 w316 w342 w365 w378 w403 w471 w482 w555 w563 w573 w602 w608] -> w119
      tunnel: [_ _ _ _ _ _ _ _ _ _ _ _ _ _ _ _ TRUE _] -> w118
      tunnel: w114 -> [_ _ _ w178 _ _ w309 _ _ _ w400 w469 _ _ w562 _ w593 _]
      tunnel: w117 -> [_ _ _ _ _ _ _ _ _ _ _ _ _ _ _ _ w598 _]
      tunnel: w110 -> [w127 _ _ _ _ _ _ _ w361 w374 _ _ _ _ _ _ w589 _]
      tunnel: [w130 w140 w152 w180 w266 dbl[] [] w314 w341 w364 w372 w399 w468 w485 w554 w557 w566 w588 w605] -> w109
      tunnel: w108 -> [w130 w140 w152 w180 w266 _ w314 w341 w364 w372 w399 w468 w485 w554 w557 w566 w588 w605]
      tunnel: [w122 w139 w151 w179 w261 w278 w313 w340 w352 w368 w398 w464 w484 w553 w556 w565 w587 w604] -> w107
      tunnel: w106 -> [w122 w139 w151 w179 w261 w278 w313 w340 _ w368 w398 w464 w484 w553 w556 w565 w587 w604]
      tunnel: w104 -> [_ _ _ _ _ _ _ _ _ _ _ _ _ _ _ _ w585 _]
      tunnel: w103 -> [_ _ _ w173 _ _ _ _ _ _ _ _ _ _ _ _ _ _]
      tunnel: w102 -> [_ _ _ _ _ _ _ _ _ _ _ _ _ _ _ _ _ _]
      tunnel: w101 -> [_ _ _ w168 _ _ _ _ _ _ _ _ _ _ _ _ _ _]
      tunnel: w99 -> [_ _ w141 _ _ _ _ _ _ _ _ _ _ _ _ _ _ _]
      frame "Initialize" {
        # "Initialize"
        n52 = Unbundle By Name(w127) -> ("Auto"=w129:refnum<queue>)
        n53 = global write "Specs.vi" "All Specs"(w122) -> ()
        n54 = call-poly "Enqueue Message.vi"("error in (no error)"=w126, "Message Data"=w122, "Message"="Update Specs", "Message Queue"=w129) -> ("error out"=w125:errorcluster)  [unwired: 6 in, 1 out]
        n55 = global write "Towerlight GV.vi" "Status"(Towerlight."Idle" ("Status")) -> ()
        n56 = control-ref of="Settings Tab Control"() -> (w121:refnum<vi>)
        n57 = control-ref of="Exit"() -> (w133:refnum<vi>)
        n58 = control-ref of="EOL"() -> (w132:refnum<vi>)
        n59 = Bundle("Exit"=w133, "EOL"=w132, "Settings Tab Control"=w121) -> (w131:T22)  [unwired: 1 in]
        "EOL" <- Main_Tabs."Home Screen" ("EOL")
      }
      frame "Manual" {
        n60 = Unbundle By Name(w136) -> ("EOL"=w138:refnum<vi>)
        n61 = property class="TabCtl (strict)"(reference=w138, error in=w135, "Value"=Main_Tabs."Manual Mode") -> (error out=w137:errorcluster)  [unwired: 1 out]
      }
      frame "Maintenance" {
        n62 = Unbundle By Name(w149) -> ("EOL"=w150:refnum<vi>)
        n63 = disable-structure shown="Enabled" {
          disable-tunnel: w141 -> [w155 _]
          frame Enabled {
            n64 = call "FGV - DO.vi"("State"=FGV_DO."Read DO") -> ("Digital Out"=w153:bool[])  [unwired: 9 in, 1 out]
            n65 = for {
              tunnel: w153 -> [w158] mode=indexing
              tunnel: w155 -> [w156] mode=indexing
              i -> [w157]
              n66 = property class="Bool (strict)"(reference=w156, "Value"=w158) -> ()  [unwired: 1 in, 2 out]
              "Numeric Control" <- w157
            }
          }
          frame Disabled {
          }
        }
        n67 = property class="TabCtl (strict)"(reference=w150, error in=w148, "Value"=Main_Tabs."Maintenance") -> (error out=w145:errorcluster)  [unwired: 1 out]
        n68 = global write "Towerlight GV.vi" "Status"(Towerlight."Maintenance" ("Status")) -> ()
        n69 = call-poly "Enqueue Message.vi"("error in (no error)"=w145, "Message"="Update Maintenance", "Message Queue"=w144) -> ("error out"=w142:errorcluster)  [unwired: 7 in, 1 out]
      }
      frame "Manual Test" {
        n70 = Variant To Data(error in=w177, type="", Variant=w178) -> (data=w175:string, error out=w161:errorcluster)
        n71 = global read "All Inputs.vi" "Input Tasks"() -> (w169:T23)
        n72 = call "SACB.vi"("Command"=enum16{"Create", "Read", "Close"}."Create", "Error In"=w161, "Model Name"="Model Name") -> ("Error Out"=w160:errorcluster)  [unwired: 6 in, 2 out]
        n73 = call <vilib>:"Acquire Semaphore.vi"("error in (no error)"=w160, "semaphore"=w168) -> ("error out"=w170:errorcluster, "semaphore out"=w171:T15)  [unwired: 3 in, 1 out]
        n74 = Not(x="Load?") -> (.not. x?=w165:bool)
        n75 = while {
          tunnel: w175 -> [w199]
          shift-right: [w196] -> _
          shift-left: TRUE ("Completed") -> [w197]
          tunnel: [w195] -> w167
          tunnel: "Model Name" -> [w192]
          tunnel: w170 -> [w189]
          tunnel: w171 -> [_]
          tunnel: w169 -> [w201]
          tunnel: w165 -> [w193]
          tunnel: "Shipping" -> [w190]
          tunnel: [enum16{"Create", "Read", "Close"}."Close" ("Command")] -> w159
          stop <- w202 stop-if-true
          n76 = call "SACB.vi"("Command"=enum16{"Create", "Read", "Close"}."Read", "Error In"=w189) -> ("Digital Inputs"=w188:T12)  [unwired: 7 in, 2 out]
          n77 = call "Auto AVG.vi"("error in"=w189, "All Input Tasks in"=w201) -> ("error out"=w198:errorcluster, "All Inputs cluster"=w187:T24)  [unwired: 7 in, 1 out]
          n78 = Bundle By Name(cluster=w187, "SACB Inputs"=w188) -> (w186:T24)
          n79 = global write "All Inputs.vi" "All Inputs"(w187) -> ()
          n80 = case shown="\"Shipping Position\"" w199 {
            tunnel: [w204 w211 w214 w225 w229 w244 w254] -> w196
            tunnel: w197 -> [w204 w207 w215 w221 w231 w240 w250]
            tunnel: [w203 w210 w217 w224 w232 w243 w253] -> w195
            tunnel: w198 -> [w203 w209 w218 w223 w233 w242 w252]
            tunnel: w186 -> [_ w208 w216 w222 w234 w241 w251]
            tunnel: w193 -> [_ _ _ _ _ w239 w249]
            tunnel: [_ w206 w213 w220 w230 w237 w248] -> w194
            tunnel: w192 -> [_ w205 w212 w219 w227 w235 w245]
            tunnel: [_ _ _ _ _ w236 w246] -> w191
            tunnel: w190 -> [_ _ _ _ w228 _ _]
            frame Default {
            }
            frame "De-Clamp" {
              n81 = call "De-Clamp.vi"("Model Name"=w205, "Error In"=w209, "Intialize?"=w207, "Inputs"=w208) -> ("error out"=w210:errorcluster, "Completed"=w211:bool, "Status"=w206:cluster{"Status":string, "Elapsed Time":dbl})  [unwired: 5 in]
            }
            frame "Clamp" {
              n82 = call "Clamp.vi"("Model Name"=w212, "Error In"=w218, "Intialize?"=w215, "Inputs"=w216) -> ("error out"=w217:errorcluster, "Completed"=w214:bool, "Status"=w213:cluster{"Status":string, "Elapsed Time":dbl})  [unwired: 5 in]
            }
            frame "Homing" {
              n83 = call "Homing.vi"("Model Name"=w219, "Error In"=w223, "Intialize?"=w221, "Inputs"=w222) -> ("error out"=w224:errorcluster, "Completed"=w225:bool, "Status"=w220:cluster{"Status":string, "Elapsed Time":dbl})  [unwired: 5 in]
            }
            frame "Shipping Position" {
              n84 = call "Shipping Position.vi"("Shipping"=w228, "Model Name"=w227, "Error In"=w233, "Intialize?"=w231, "Inputs"=w234) -> ("error out"=w232:errorcluster, "Completed"=w229:bool, "Results"=→"Shipping":cluster{"Shipping Position":dbl}, "Status"=w230:cluster{"Status":string, "Elapsed Time":dbl})  [unwired: 3 in]
            }
            frame "Go Up" {
              n85 = call "Go UP (Loaded).vi"("Skip Loading?"=w239, "Model Name"=w235, "Error In"=w242, "Intialize?"=w240, "Inputs"=w241) -> ("error out"=w243:errorcluster, "Completed"=w244:bool, "Results"=→"GO UP":T25, "Status"=w237:cluster{"Status":string, "Elapsed Time":dbl}, "Graph"=w236:dbl[][])  [unwired: 2 in]
            }
            frame "Go Down" {
              n86 = call "Go Down (Loaded).vi"("Skip Load?"=w249, "Model Name"=w245, "Error In"=w252, "Intialize?"=w250, "Inputs"=w251) -> ("error out"=w253:errorcluster, "Completed"=w254:bool, "Results"=→"GO DOWN":T26, "Status"=w248:cluster{"Status":string, "Elapsed Time":dbl}, "Array"=w246:dbl[][])  [unwired: 2 in]
            }
          }
          "StatusManual" <- w194
          "Manual Graph" <- w191
          "manual error" <- w195
          n87 = Wait Until Next ms Multiple(millisecond multiple=u32 20 ("milliseconds to wait")) -> ()  [unwired: 1 out]
          n88 = Compound Arithmetic op=OR(w196, w195) -> (w202:bool)
        }
        n89 = global write "Specs.vi" "Shipping"("Shipping") -> ()
        n90 = for {
          tunnel: w173 -> [w183] mode=indexing
          tunnel: T18."Enabled" ("Disabled") -> [w182]
          tunnel: w167 -> [_]
          n91 = property class="Bool"(reference=w183, "DisabledEnum"=w182) -> ()  [unwired: 1 in, 2 out]
        }
        n92 = call <vilib>:"Release Semaphore.vi"("error in (no error)"=w167, "semaphore"=w168) -> ()  [unwired: 4 in, 2 out]
        n93 = call "SACB.vi"("Command"=w159) -> ()  [unwired: 8 in, 3 out]
      }
      frame "Calibration" {
        n94 = Unbundle By Name(w269) -> ("EOL"=w268:refnum<vi>)
        n95 = for {
          tunnel: tag[] ["1922_LoadCell", "1922_CurrentMon", "1922_Stroke"] -> [w273] mode=indexing
          tunnel: [w270] -> w259 mode=indexing
          n96 = property class="DAQmx Scale"("Active Scale"=w273) -> ("Lin.Slope"=w272:dbl, "Lin.YIntercept"=w271:dbl)  [unwired: 2 in, 2 out]
          n97 = Bundle("Lin.Slope"=w272, "Lin.YIntercept"=w271) -> (w270:cluster{"Lin.Slope":dbl, "Lin.YIntercept":dbl})  [unwired: 1 in]
        }
        n98 = property class="TabCtl (strict)"(reference=w268, error in=w267, "Value"=Main_Tabs."Calibration") -> (error out=w262:errorcluster)  [unwired: 1 out]
        n99 = Index Array(array=w259) -> (element #1=w258:cluster{"Lin.Slope":dbl, "Lin.YIntercept":dbl}, element #2=w257:cluster{"Lin.Slope":dbl, "Lin.YIntercept":dbl}, element #3=w255:cluster{"Lin.Slope":dbl, "Lin.YIntercept":dbl})  [unwired: 3 in]
        n100 = local write "Load Cell"(w258) -> ()
        n101 = local write "Stroke Sensor"(w255) -> ()
        n102 = local write "Current"(w257) -> ()
        n103 = call-poly "Enqueue Message.vi"("error in (no error)"=w262, "Message"="Update Calibrate", "Message Queue"=w264) -> ("error out"=w265:errorcluster)  [unwired: 7 in, 1 out]
      }
      frame "Update Calibrate" {
        # "Update Calibration Table"
        n104 = for {
          tunnel: tag[] ["1922_LoadCell", "1922_CurrentMon", "1922_Stroke"] -> [w279] mode=indexing
          i -> [w283]
          n105 = case shown="1" w283 {
            tunnel: [w286 w289 w292] -> w282
            tunnel: [w285 w288 w291] -> w281
            frame 0, Default {
              n106 = Unbundle By Name("Load Cell") -> ("Slope"=w286:dbl, "Intercept"=w285:dbl)
            }
            frame 1 {
              n107 = Unbundle By Name("Current") -> ("Slope"=w289:dbl, "Intercept"=w288:dbl)
            }
            frame 2 {
              n108 = Unbundle By Name("Stroke Sensor") -> ("Slope"=w292:dbl, "Intercept"=w291:dbl)
            }
          }
          n109 = property class="DAQmx Scale"("Active Scale"=w279, "Lin.Slope"=w282, "Lin.YIntercept"=w281) -> (error out=w280:errorcluster)  [unwired: 2 in, 1 out]
          n110 = call <vilib>:"DAQmx Save Scale.vi"("scale name"=w279, "error in"=w280) -> ()  [unwired: 13 in, 1 out]
        }
      }
      frame "Settings" {
        n111 = Unbundle By Name(w316) -> ("EOL"=w315:refnum<vi>, "Settings Tab Control"=w301:refnum<vi>)
        n112 = Variant To Data(error in=w308, type=T10."LH" ("Settings Mode Change"), Variant=w309) -> (data=w306:T10, error out=w307:errorcluster)
        n113 = Unbundle By Name(w313) -> ("LH"=w311:T2, "RH"=w310:T2, "W 601 FR RH Std"=w304:T2, "W 601 FR LH Std"=w303:T2, "W 601 RR RH Std"=w302:T2, "W 601 RR LH Std"=w297:T2, "W 601 FR RH AP"=w296:T2, "W 601 FR LH AP"=w295:T2, "W 601 RR RH AP"=w294:T2, "W 601 RR LH AP"=w293:T2)
        n114 = property class="TabCtl (strict)"(reference=w315, error in=w307, "Value"=Main_Tabs."Settings") -> (error out=w299:errorcluster)  [unwired: 1 out]
        n115 = case shown="\"W 601 RR LH AP\"" w306 {
          tunnel: [T10."LH" ("Value") T10."RH" ("Value") T10."W 601 FR RH Std" ("Value") T10."W 601 FR LH Std" ("Value") T10."W 601 RR RH Std" ("Value") T10."W 601 RR LH Std" ("Value") T10."W 601 FR RH AP" ("Value") T10."W 601 FR LH AP" ("Value") T10."W 601 RR RH AP" ("Value") T10."W 601 RR LH AP" ("Value")] -> w300
          frame "LH", Default {
          }
          frame "RH" {
          }
          frame "W 601 FR RH Std" {
          }
          frame "W 601 FR LH Std" {
          }
          frame "W 601 RR RH Std" {
          }
          frame "W 601 RR LH Std" {
          }
          frame "W 601 FR RH AP" {
          }
          frame "W 601 FR LH AP" {
          }
          frame "W 601 RR RH AP" {
          }
          frame "W 601 RR LH AP" {
          }
        }
        n116 = local write "LH"(w311) -> ()
        n117 = local write "RH"(w310) -> ()
        n118 = local write "W 601 FR RH Std"(w304) -> ()
        n119 = local write "W 601 FR LH Std"(w303) -> ()
        n120 = local write "W 601 RR RH Std"(w302) -> ()
        n121 = local write "W 601 RR LH Std"(w297) -> ()
        n122 = local write "W 601 FR RH AP"(w296) -> ()
        n123 = local write "W 601 FR LH AP"(w295) -> ()
        n124 = local write "W 601 RR RH AP"(w294) -> ()
        n125 = local write "W 601 RR LH AP"(w293) -> ()
        n126 = property class="TabCtl (strict)"(reference=w301, error in=w299, "Value"=w300) -> (error out=w298:errorcluster)  [unwired: 1 out]
      }
      frame "Test Print" {
        n127 = Format Date/Time String(time format string (%c)="%d-%m-%Y") -> (date/time string=w329:string)  [unwired: 2 in]
        n128 = Format Date/Time String(time format string (%c)="%H:%M:%S") -> (date/time string=w328:string)  [unwired: 2 in]
        n129 = Concatenate Strings(w329, " " ("string"), w328) -> ()  [unwired: 1 out]
        n130 = Build Array (concatenate)(string[] [" ", " "] ("PrintPara"), "Part Number", "Part Name", "ID", "Shift", w329, w328, "Number") -> (w338:string[])
        n131 = call "PrintLabel v0.4.vi"("PrintPara"=w338) -> ()  [unwired: 10 in, 1 out]
      }
      frame "Save Specs" {
        n132 = Unbundle By Name(w361) -> ("Auto"=w363:refnum<queue>)
        n133 = Bundle By Name(cluster=T1 {"LH"={"Go Up"={"Min Speed"=120.0, "Max Speed"=10.0, "Min Time"=1.82, "Max Time"=3.7, "Min Run Current"=0.0, "Max Run Current"=10.0, "Min Stall Current"=0.0, "Max Stall Current"=25.0, "Min Stall Force"=170.0, "Max Stall Force"=320.0, "Min Stroke"=170.0, "Max Stroke"=320.0}, "Go Down"={"Min Speed"=10.0, "Max Speed"=250.0, "Min Travel Time"=1.82, "Max Travel Time"=3.7, "Min Run Current"=0.0, "Max Run Current"=10.0}, "Shipping"={"Min Distance"=150.0, "Max Distance"=300.0, "Setpoint"=5.0}, "Anti-Pinch"={"Min Force"=5.0, "Max Force"=15.0}}, "RH"={"Go Up"={"Min Speed"=120.0, "Max Speed"=10.0, "Min Time"=1.82, "Max Time"=3.7, "Min Run Current"=0.0, "Max Run Current"=10.0, "Min Stall Current"=0.0, "Max Stall Current"=25.0, "Min Stall Force"=170.0, "Max Stall Force"=320.0, "Min Stroke"=170.0, "Max Stroke"=320.0}, "Go Down"={"Min Speed"=10.0, "Max Speed"=250.0, "Min Travel Time"=1.82, "Max Travel Time"=3.7, "Min Run Current"=0.0, "Max Run Current"=10.0}, "Shipping"={"Min Distance"=150.0, "Max Distance"=300.0, "Setpoint"=5.0}, "Anti-Pinch"={"Min Force"=5.0, "Max Force"=15.0}}, "W 601 FR RH Std"={"Go Up"={"Min Speed"=10.0, "Max Speed"=250.0, "Min Time"=0.5, "Max Time"=4.3, "Min Run Current"=0.0, "Max Run Current"=10.0, "Min Stall Current"=0.0, "Max Stall Current"=25.0, "Min Stall Force"=170.0, "Max Stall Force"=320.0, "Min Stroke"=254.4, "Max Stroke"=270.4}, "Go Down"={"Min Speed"=10.0, "Max Speed"=250.0, "Min Travel Time"=0.5, "Max Travel Time"=4.3, "Min Run Current"=0.0, "Max Run Current"=10.0}, "Shipping"={"Min Distance"=5.0, "Max Distance"=15.0, "Setpoint"=5.0}, "Anti-Pinch"={"Min Force"=5.0, "Max Force"=15.0}}, "W 601 FR LH Std"={"Go Up"={"Min Speed"=10.0, "Max Speed"=250.0, "Min Time"=0.5, "Max Time"=4.3, "Min Run Current"=0.0, "Max Run Current"=10.0, "Min Stall Current"=0.0, "Max Stall Current"=25.0, "Min Stall Force"=170.0, "Max Stall Force"=320.0, "Min Stroke"=254.4, "Max Stroke"=270.4}, "Go Down"={"Min Speed"=10.0, "Max Speed"=250.0, "Min Travel Time"=0.5, "Max Travel Time"=4.3, "Min Run Current"=0.0, "Max Run Current"=10.0}, "Shipping"={"Min Distance"=5.0, "Max Distance"=15.0, "Setpoint"=5.0}, "Anti-Pinch"={"Min Force"=5.0, "Max Force"=15.0}}, "W 601 RR RH Std"={"Go Up"={"Min Speed"=10.0, "Max Speed"=250.0, "Min Time"=0.5, "Max Time"=4.3, "Min Run Current"=0.0, "Max Run Current"=10.0, "Min Stall Current"=0.0, "Max Stall Current"=25.0, "Min Stall Force"=170.0, "Max Stall Force"=320.0, "Min Stroke"=254.4, "Max Stroke"=270.4}, "Go Down"={"Min Speed"=10.0, "Max Speed"=250.0, "Min Travel Time"=0.5, "Max Travel Time"=4.3, "Min Run Current"=0.0, "Max Run Current"=10.0}, "Shipping"={"Min Distance"=5.0, "Max Distance"=15.0, "Setpoint"=5.0}, "Anti-Pinch"={"Min Force"=5.0, "Max Force"=15.0}}, "W 601 RR LH Std"={"Go Up"={"Min Speed"=10.0, "Max Speed"=250.0, "Min Time"=0.5, "Max Time"=4.3, "Min Run Current"=0.0, "Max Run Current"=10.0, "Min Stall Current"=0.0, "Max Stall Current"=25.0, "Min Stall Force"=170.0, "Max Stall Force"=320.0, "Min Stroke"=254.4, "Max Stroke"=270.4}, "Go Down"={"Min Speed"=10.0, "Max Speed"=250.0, "Min Travel Time"=0.5, "Max Travel Time"=4.3, "Min Run Current"=0.0, "Max Run Current"=10.0}, "Shipping"={"Min Distance"=5.0, "Max Distance"=15.0, "Setpoint"=5.0}, "Anti-Pinch"={"Min Force"=5.0, "Max Force"=15.0}}, "W 601 FR RH AP"={"Go Up"={"Min Speed"=10.0, "Max Speed"=250.0, "Min Time"=0.5, "Max Time"=4.3, "Min Run Current"=0.0, "Max Run Current"=10.0, "Min Stall Current"=0.0, "Max Stall Current"=25.0, "Min Stall Force"=170.0, "Max Stall Force"=320.0, "Min Stroke"=254.4, "Max Stroke"=270.4}, "Go Down"={"Min Speed"=10.0, "Max Speed"=250.0, "Min Travel Time"=0.5, "Max Travel Time"=4.3, "Min Run Current"=0.0, "Max Run Current"=10.0}, "Shipping"={"Min Distance"=5.0, "Max Distance"=15.0, "Setpoint"=5.0}, "Anti-Pinch"={"Min Force"=5.0, "Max Force"=15.0}}, "W 601 FR LH AP"={"Go Up"={"Min Speed"=10.0, "Max Speed"=250.0, "Min Time"=0.5, "Max Time"=4.3, "Min Run Current"=0.0, "Max Run Current"=10.0, "Min Stall Current"=0.0, "Max Stall Current"=25.0, "Min Stall Force"=170.0, "Max Stall Force"=320.0, "Min Stroke"=254.4, "Max Stroke"=270.4}, "Go Down"={"Min Speed"=10.0, "Max Speed"=250.0, "Min Travel Time"=0.5, "Max Travel Time"=4.3, "Min Run Current"=0.0, "Max Run Current"=10.0}, "Shipping"={"Min Distance"=5.0, "Max Distance"=15.0, "Setpoint"=5.0}, "Anti-Pinch"={"Min Force"=5.0, "Max Force"=15.0}}, "W 601 RR RH AP"={"Go Up"={"Min Speed"=10.0, "Max Speed"=250.0, "Min Time"=0.5, "Max Time"=4.3, "Min Run Current"=0.0, "Max Run Current"=10.0, "Min Stall Current"=0.0, "Max Stall Current"=25.0, "Min Stall Force"=170.0, "Max Stall Force"=320.0, "Min Stroke"=254.4, "Max Stroke"=270.4}, "Go Down"={"Min Speed"=10.0, "Max Speed"=250.0, "Min Travel Time"=0.5, "Max Travel Time"=4.3, "Min Run Current"=0.0, "Max Run Current"=10.0}, "Shipping"={"Min Distance"=5.0, "Max Distance"=15.0, "Setpoint"=5.0}, "Anti-Pinch"={"Min Force"=5.0, "Max Force"=15.0}}, "W 601 RR LH AP"={"Go Up"={"Min Speed"=10.0, "Max Speed"=250.0, "Min Time"=0.5, "Max Time"=4.3, "Min Run Current"=0.0, "Max Run Current"=10.0, "Min Stall Current"=0.0, "Max Stall Current"=25.0, "Min Stall Force"=170.0, "Max Stall Force"=320.0, "Min Stroke"=254.4, "Max Stroke"=270.4}, "Go Down"={"Min Speed"=10.0, "Max Speed"=250.0, "Min Travel Time"=0.5, "Max Travel Time"=4.3, "Min Run Current"=0.0, "Max Run Current"=10.0}, "Shipping"={"Min Distance"=5.0, "Max Distance"=15.0, "Setpoint"=5.0}, "Anti-Pinch"={"Min Force"=5.0, "Max Force"=15.0}}} ("All Specs"), "LH"="LH", "RH"="RH", "W 601 FR RH Std"="W 601 FR RH Std", "W 601 FR LH Std"="W 601 FR LH Std", "W 601 RR RH Std"="W 601 RR RH Std", "W 601 RR LH Std"="W 601 RR LH Std", "W 601 FR RH AP"="W 601 FR RH AP", "W 601 FR LH AP"="W 601 FR LH AP", "W 601 RR RH AP"="W 601 RR RH AP", "W 601 RR LH AP"="W 601 RR LH AP") -> (w352:T1)
        n134 = call <vilib>:"Application Directory.vi"() -> ("Application Directory"=w353:path)
        n135 = call-poly "Enqueue Message.vi"("error in (no error)"=w360, "Message Data"=w352, "Message"="Update Specs", "Message Queue"=w363) -> ("error out"=w355:errorcluster)  [unwired: 6 in, 1 out]
        n136 = Build Path(base path=w353, name or relative path="config.ini") -> (appended path=w356:path)
        n137 = global write "Specs.vi" "All Specs"(w352) -> ()
        n138 = call "Write Config.vi"("error in (no error)"=w355, "output cluster"=w352, "file path"=w356) -> ("error out"=w354:errorcluster)  [unwired: 7 in, 1 out]
      }
      frame "Autocycle" {
        n139 = Unbundle By Name(w374) -> ("Auto"=w373:refnum<queue>)
        n140 = call "Select Model.vi"() -> ("Cancelled"=w370:bool, "Initial Data"=w366:T27)  [unwired: 10 in]
        n141 = global write "Specs.vi" "All Specs"(w368) -> ()
        n142 = Unbundle By Name(w366) -> ("Model Name"=w369:T9)
        n143 = case shown="\"W 501 FLH Std.\", Default" w369 {
          tunnel: w368 -> [w380 w382 _ _ _ _ _ _ _ _]
          tunnel: [w379 w381 _ _ _ _ _ _ _ _] -> w367
          frame "W 501 FLH Std.", Default {
            n144 = Unbundle By Name(w380) -> ("LH.Shipping.Setpoint"=w379:dbl)
          }
          frame "W 501 FRH Std." {
            n145 = Unbundle By Name(w382) -> ("RH.Shipping.Setpoint"=w381:dbl)
          }
          frame "W 601 FR RH Std" {
          }
          frame "W 601 FR LH Std" {
          }
          frame "W 601 RR RH Std" {
          }
          frame "W 601 RR LH Std" {
          }
          frame "W 601 FR RH AP" {
          }
          frame "W 601 FR LH AP" {
          }
          frame "W 601 RR RH AP" {
          }
          frame "W 601 RR LH AP" {
          }
        }
        n146 = Format Into String(w369) -> (resulting string=→"Model Name 2":string)  [unwired: 3 in, 1 out]
        n147 = Unbundle By Name(w378) -> ("EOL"=w377:refnum<vi>)
        n148 = case shown="False" w370 {
          tunnel: w377 -> [w391 _]
          tunnel: [w390 w392] -> w376
          tunnel: w375 -> [w389 w392]
          tunnel: w373 -> [w387 _]
          tunnel: w366 -> [w384 _]
          frame False {
            n149 = call-poly "Enqueue Message.vi"("error in (no error)"=w389, "Message Data"=w384, "Message"="Start Auto Mode", "Message Queue"=w387) -> ("error out"=w388:errorcluster)  [unwired: 6 in, 1 out]
            n150 = property on="Results" class="Clust (strict)"("Blinking"=FALSE) -> ()  [unwired: 2 in, 2 out]
            n151 = property class="TabCtl (strict)"(reference=w391, error in=w388, "Value"=Main_Tabs."Autocycle") -> (error out=w390:errorcluster)  [unwired: 1 out]
          }
          frame True {
          }
        }
        n152 = global write "Specs.vi" "Shipping"(w367) -> ()
      }
      frame "Update Status" {
        # "Update Measurements"
        n153 = Variant To Data(error in=w402, type=Auto_States_v0.2."Initialize" ("AC State"), Variant=w400) -> (data=w396:T19, error out=w401:errorcluster)
        n154 = case shown="\"Wait for Part Presence\"" w396 {
          selector: w396 -> [_ _ _ _ _ _ _ _ w447 w451]
          tunnel: [Towerlight."Idle" ("Status") Towerlight."Idle" ("Status") Towerlight."Idle" ("Status") Towerlight."Idle" ("Status") Towerlight."Idle" ("Status") Towerlight."Idle" ("Status") Towerlight."Running" ("Status") Towerlight."Idle" ("Status") Towerlight."Idle" ("Status") Towerlight."Idle" ("Status")] -> w397
          tunnel: ["Incoming Air Pressure Not OK" "E-Stop is Pressed" "Please Close the Reject Door" "Press Start to Begin Homing" "Please load the Part" "Press Start to Start the Test" w428 w441 w446 w450] -> w395
          tunnel: [u16 5 ("AC Pictures") u16 4 ("AC Pictures") u16 4 ("AC Pictures") u16 8 ("AC Pictures") u16 6 ("AC Pictures") u16 7 ("AC Pictures") u16 3 ("AC Pictures") w434 u16 9 ("AC Pictures") _] -> w394
          frame "Check Pressure" {
          }
          frame "Check EStop" {
          }
          frame "Check ReadyCondition" {
          }
          frame "Wait to Home" {
            n155 = property on="Results" class="Clust (strict)"("Blinking"=FALSE) -> ()  [unwired: 2 in, 2 out]
          }
          frame "Wait for Part Presence" {
            n156 = property on="Results" class="Clust (strict)"("Blinking"=FALSE) -> ()  [unwired: 2 in, 2 out]
          }
          frame "Wait for Start" {
            n157 = property on="Results" class="Clust (strict)"("Blinking"=FALSE) -> ()  [unwired: 2 in, 2 out]
          }
          frame "Test Sequencer" {
            n158 = local read "TS Status"() -> (w429:cluster{"Status":string, "Elapsed Time":dbl})
            n159 = Unbundle By Name(w429) -> ("Status"=w427:string)
            n160 = Concatenate Strings("Testing in Progress: (", w427, ")" ("string")) -> (w428:string)
          }
          frame "Result" {
            n161 = local read "Results"() -> (w440:T5)
            n162 = Unbundle By Name(w440) -> ("Results.PASS?"=w432:bool)
            n163 = Select(t="PASS", s=w432, f="FAIL") -> (s? t:f=w437:string)
            n164 = case shown="True" w432 {
              frame True {
              }
              frame False {
                n165 = property on="Results" class="Clust (strict)"("Blinking"=TRUE) -> ()  [unwired: 2 in, 2 out]
              }
            }
            n166 = Concatenate Strings("Test Result: ", w437, " (Unload Part)" ("string")) -> (w441:string)
            n167 = Select(t=u16 2 ("AC Pictures"), s=w432, f=u16 1 ("AC Pictures")) -> (s? t:f=w434:u16)
          }
          frame "Wait for Reject Door Open".."Wait for Reject Door Close" {
            n168 = Format Into String(w447) -> (resulting string=w446:string)  [unwired: 3 in, 1 out]
          }
          frame Default {
            n169 = Format Into String(w451) -> (resulting string=w450:string)  [unwired: 3 in, 1 out]
            n170 = property on="Results" class="Clust (strict)"("Blinking"=FALSE) -> ()  [unwired: 2 in, 2 out]
          }
        }
        "Status" <- w395
        "AC Pictures" <- w394
        n171 = global write "Towerlight GV.vi" "Status"(w397) -> ()
      }
      frame "Update Measurements" {
        # "Update Measurements"
        n172 = Variant To Data(error in=w470, type=T20 {"Results"={"Initial"={"Date"="", "Time"="", "ID"=""}, "Go Up"={"Speed"=0.0, "Travel Time"=0.0, "Running Current"=0.0, "Up Stroke"=0.0, "Stall Current"=0.0, "Stall Force"=0.0}, "Go Down"={"Speed"=0.0, "Travel Time"=0.0, "Running Current"=0.0, "Down Stroke"=0.0}, "Shipping Position"={"Shipping Position"=0.0}, "Results"={"PASS?"=FALSE, "Details"=""}}, "TS Status"={"Status"="", "Elapsed Time"=0.0}, "Counts"={"TotalCount"=0, "PassCount"=0, "FailCount"=0}, "AC Graph"=[], "Total Time"=0.0, "Testing Time (s)"=0.0, "Graph"=[], "signal out"={"t0"=timestamp(0 s since 1904-01-01), "dt"=1.0, "Y"=[]}} ("cluster"), Variant=w469) -> (data=w466:T20, error out=w463:errorcluster)
        n173 = Unbundle By Name(w466) -> ("Total Time"=→"Total Time":dbl, "Testing Time (s)"=w454:dbl, "Results"=→"Results":T5, "TS Status"=→"TS Status":cluster{"Status":string, "Elapsed Time":dbl}, "Counts"=→"Counts":T6, "Graph"=w459:dbl[][])
        n174 = Index Array(array=w459) -> (element #1=w458:dbl[], element #2=w457:dbl[])  [unwired: 4 in]
        n175 = Divide(x=w454, y=1000.0) -> (x/y=→"Testing Time (s)":dbl)
        n176 = Bundle("Graph"=w458, "Graph"=w457) -> (→"AC Graph":cluster{"Graph":dbl[], "Graph":dbl[]})  [unwired: 1 in]
      }
      frame "Update Maintenance" {
        # "Update Measurements"
        n177 = global read "All Inputs.vi" "SACB Connection"() -> (w473:i32)
        n178 = Unbundle By Name(w482) -> ("EOL"=w481:refnum<vi>)
        n179 = global read "All Inputs.vi" "All Inputs"() -> (w479:T24)
        n180 = property class="TabCtl (strict)"(reference=w481) -> ("Value"=w480:T3)  [unwired: 1 in, 2 out]
        n181 = Greater Or Equal To 0?(x=w473) -> (x >= 0?=w472:bool)
        n182 = case shown="\"Maintenance\"" w480 {
          tunnel: w479 -> [_ w513]
          tunnel: "Reset Graph" -> [_ w524]
          tunnel: "Average" -> [_ w500]
          tunnel: w478 -> [w487 w520]
          tunnel: w477 -> [_ w519]
          tunnel: [w487 w518] -> w476
          tunnel: "Pause" -> [_ w498]
          tunnel: w472 -> [_ w488]
          frame Default {
            # "Automatically stops when tab has changed to Home"
            n183 = global write "Towerlight GV.vi" "Status"(Towerlight."Idle" ("Status")) -> ()
          }
          frame "Maintenance" {
            n184 = Unbundle By Name(w513) -> ("AI.Force"=w522:dbl[], "AI.Stroke"=w525:dbl[], "AI.CurrentMon"=w523:dbl[], "DI.Machine ON"=→"Machine ON":bool, "DI.E-Stop"=→"E-Stop":bool, "DI.Pressure"=→"Pressure":bool, "DI.Start"=→"Start":bool, "DI.Safety Curtain"=→"Safety Curtain":bool, "DI.RS Load UP Rear"=→"RS Load UP Rear":bool, "DI.RS Load UP Front"=→"RS Load UP Front":bool, "DI.RS Load DN Rear"=→"RS Load DN Rear":bool, "DI.RS Load DN Front"=→"RS Load DN Front":bool, "DI.RS Loadcell Rear"=→"RS Loadcell Rear":bool, "DI.RS Loadcell Front"=→"RS Loadcell Front":bool, "DI.Reject Sensor 1"=→"Reject Sensor 1":bool, "DI.Reject Sensor 2"=→"Reject Sensor 2":bool, "DI.Door SW Reject"=→"Reject Door SW":bool)
            n185 = case shown="True" w488 {
              tunnel: [_ w528] -> w490
              tunnel: [_ w526] -> w489
              frame False {
              }
              frame True {
                n186 = call "SACB.vi"("Command"=enum16{"Create", "Read", "Close"}."Read") -> ("Connected?"=w528:bool, "Digital Inputs"=w526:T12)  [unwired: 8 in, 1 out]
              }
            }
            "SACB Inputs" <- w489
            "Connected?" <- w490
            n187 = case shown="False" w500 {
              tunnel: [w538 w548] -> w516
              tunnel: w522 -> [w537 w544]
              tunnel: w525 -> [w536 w543]
              tunnel: [w535 w547] -> w514
              tunnel: w524 -> [w532 w545]
              tunnel: w523 -> [w534 w542]
              tunnel: [w533 w546] -> w515
              tunnel: [w531 w539] -> w495
              tunnel: [w530 w540] -> w494
              tunnel: [w529 w541] -> w493
              frame True {
                n188 = call "Array Average.vi"("data"=w537) -> ("Numeric"=w529:dbl)  [unwired: 10 in]
                n189 = call "Array Average.vi"("data"=w536) -> ("Numeric"=w530:dbl)  [unwired: 10 in]
                n190 = call "Array Average.vi"("data"=w534) -> ("Numeric"=w531:dbl)  [unwired: 10 in]
                n191 = call "Build Graph.vi"("Numeric"=w529, "Reset Graph"=w532) -> ("Array"=w535:dbl[])  [unwired: 9 in]
                n192 = call "Build Graph.vi"("Numeric"=w530, "Reset Graph"=w532) -> ("Array"=w538:dbl[])  [unwired: 9 in]
                n193 = call "Build Graph.vi"("Numeric"=w531, "Reset Graph"=w532) -> ("Array"=w533:dbl[])  [unwired: 9 in]
              }
              frame False {
                n194 = call "Array Average.vi"("data"=w544) -> ("Numeric"=w541:dbl)  [unwired: 10 in]
                n195 = call "Array Average.vi"("data"=w543) -> ("Numeric"=w540:dbl)  [unwired: 10 in]
                n196 = call "Array Average.vi"("data"=w542) -> ("Numeric"=w539:dbl)  [unwired: 10 in]
                n197 = call "Build Graph (arr).vi"("Array in"=w544, "Reset Graph"=w545) -> ("Array"=w547:dbl[])  [unwired: 9 in]
                n198 = call "Build Graph (arr).vi"("Array in"=w543, "Reset Graph"=w545) -> ("Array"=w548:dbl[])  [unwired: 9 in]
                n199 = call "Build Graph (arr).vi"("Array in"=w542, "Reset Graph"=w545) -> ("Array"=w546:dbl[])  [unwired: 9 in]
              }
            }
            "Load Cell (N)" <- w493
            "Stroke (mm)" <- w494
            "Current (A)" <- w495
            n200 = feedback #1() -> (w497:dbl[][])  [unwired: 1 in]
            n201 = Build Array(w514, w516, w515) -> (w496:dbl[][])
            n202 = call-poly "Enqueue Message.vi"("error in (no error)"=w520, "Message"="Update Maintenance", "Message Queue"=w519) -> ("error out"=w518:errorcluster)  [unwired: 7 in, 1 out]
            n203 = Select(t=w497, s=w498, f=w496) -> (s? t:f=w492:dbl[][])
            "Graph" <- w492
            n204 = feedback-in #1(w492) -> ()
            n205 = Wait (ms)(milliseconds to wait=u32 50) -> ()  [unwired: 1 out]
          }
        }
      }
      frame "Exit Maintenance" {
        n206 = call-poly "Enqueue Message.vi"("error in (no error)"=w551, "Message"="Initialize", "Message Queue"=w549) -> ("error out"=w550:errorcluster)  [unwired: 7 in, 1 out]
      }
      frame "Error" {
        # "Error - Display an error dialog. This message is sent by the \"Error Handler\" VIs at the end of other loops in this application."
        n207 = Variant To Data(error in=w564, type=errorcluster {"status"=FALSE, "code"=0, "source"=""} ("error constant"), Variant=w562) -> (data=w560:errorcluster, error out=w559:errorcluster)
        n208 = call <vilib>:"Simple Error Handler.vi"("error in (no error)"=w560) -> ()  [unwired: 4 in, 5 out]
        n209 = Merge Errors(w559) -> (w558:errorcluster)
      }
      frame "Confirm Quit" {
        # "Confirm Quit - Message that can confirm whether or not the user wants to exit the application."
        n210 = Two Button Dialog(message="Are you sure you want to quit?", 2:"Yes" ("T button name (\"OK\")")) -> (T button?=w567:bool)  [unwired: 1 in]
        n211 = case shown="False" w567 {
          tunnel: w574 -> [w575 w580]
          tunnel: [w575 w579] -> w571
          tunnel: w570 -> [_ w578]
          frame False {
          }
          frame True {
            n212 = call-poly "Enqueue Message.vi"("Priority Message? (F)"=TRUE, "error in (no error)"=w580, "Message"="Exit", "Message Queue"=w578) -> ("error out"=w579:errorcluster)  [unwired: 6 in, 1 out]
          }
        }
        n213 = Merge Errors(w571) -> (w572:errorcluster)
      }
      frame "Exit" {
        # "Stop the VI"
        # "Release the message queue reference"
        # "Exit - Exit the application."
        n214 = Variant To Data(type=errorcluster {"status"=FALSE, "code"=0, "source"=""} ("error constant"), Variant=w593) -> (data=w594:errorcluster)  [unwired: 1 in, 1 out]
        n215 = call <vilib>:"Simple Error Handler.vi"("error in (no error)"=w594) -> ()  [unwired: 4 in, 5 out]
        n216 = Send Notification(notification=TRUE, notifier=w585) -> ()  [unwired: 1 in, 2 out]
        n217 = Release Queue(queue=w603, error in (no error)=w596) -> (error out=w600:errorcluster)  [unwired: 1 in, 2 out]
        n218 = Unbundle By Name(w589) -> ("Auto"=w592:refnum<queue>)
        n219 = call "Fire User Event - Stop.vi"("User Event - Stop"=w598) -> ("error out"=w597:errorcluster)  [unwired: 10 in]
        n220 = call "FGV - AO.vi"("State"=FGV_AO."Clear Tasks") -> ("error out"=w581:errorcluster)  [unwired: 10 in]
        n221 = call "FGV - DO.vi"("State"=FGV_DO."Clear Tasks") -> ("error out"=w586:errorcluster)  [unwired: 9 in, 1 out]
        n222 = call-poly "Enqueue Message.vi"("Message"="Exit", "Message Queue"=w592) -> ("error out"=w590:errorcluster)  [unwired: 8 in, 1 out]
        n223 = Merge Errors(w581, w586, w590, w597, w600) -> (w599:errorcluster)
      }
      frame Default {
        # "'Default' case only runs if there is a message that isn't defined in any of the other cases.  Output a programming error."
        n224 = xnode "Error Ring"("parameter 0"=w606) -> ("error out"=w607:errorcluster)
      }
    }
    n225 = call "Error Handler - Message Handling Loop.vi"("error in (no error)"=w111, "Message Queue"=w105) -> ("dup error in"=w112:errorcluster)  [unwired: 8 in, 1 out]
  }
  n226 = while {
    tunnel: w75 -> [w627]
    shift-right: [w625] -> w71
    shift-left: w68 -> [w626]
    tunnel: [w621] -> w69
    tunnel: w64 -> [w619]
    tunnel: w36 -> [w618]
    tunnel: w34 -> [w617]
    tunnel: w2 -> [w616]
    stop <- w623 stop-if-true
    # "Event Handling Loop"
    n227 = event shown="[8] \"Home Maint\": Value Change" {
      selector: w626 -> [_ _ _ _ _ _ _ _ _ _ _ _ _ _ _ _ _ _ _]
      dyn-events: [_ _ _ _ _ _ _ _ _ _ _ _ _ _ _ _ _ _ _] -> w625
      timeout: 500 -> [_ _ _ _ _ _ _ _ _ _ _ _ _ _ _ _ _ _ _]
      tunnel: [_ _ _ _ _ _ _ _ _ _ _ _ _ _ _ _ _ _ TRUE ("Discard?")] -> w623
      tunnel: w627 -> [w632 w636 w639 w651 w664 w666 w673 w679 w683 w701 w711 w718 w721 w729 w733 w737 w740 w745 w747]
      tunnel: [w631 _ w637 w649 w659 _ w671 w677 w681 _ _ _ w719 w727 w731 w735 _ w744 _] -> w624
      tunnel: [w630 w636 w638 w650 w663 w666 w672 w678 w682 w701 w711 w718 w720 w728 w732 w736 w740 w743 w747] -> w622
      tunnel: w619 -> [_ _ _ _ _ _ _ _ _ _ _ _ _ w724 _ _ _ _ _]
      tunnel: w618 -> [_ _ _ _ _ _ w668 _ _ _ _ _ _ _ _ _ _ _ _]
      tunnel: w617 -> [_ _ _ w645 _ _ _ _ _ _ _ _ _ _ _ _ _ _ _]
      tunnel: w616 -> [_ _ _ _ w660 _ _ _ _ _ _ _ _ _ _ _ _ _ _]
      event Panel Close? {
        # "Send the 'Confirm Quit' message if the user closes the panel of the VI. Discard the event so the 'Confirm Quit' message has a chance to run."
        n228 = event-data() -> ()  [unwired: 1 in, 1 out]
        n229 = call-poly "Enqueue Message.vi"("Priority Message? (F)"=TRUE, "Message"="Confirm Quit", "Message Queue"=w632) -> ("error out"=w631:errorcluster, "dup Message Queue"=w630:refnum<queue>)  [unwired: 7 in]
        n230 = event-data("Discard?"=TRUE) -> ()  [unwired: 1 in, 1 out]
      }
      event Timeout {
        n231 = event-data() -> ()  [unwired: 1 in, 1 out]
        n232 = Format Date/Time String(time format string (%c)="%d %B %Y | %I:%M:%S %p") -> (date/time string=→"String":string)  [unwired: 2 in]
      }
      event "Manual", "Calibration", "Maintenance": Value Change {
        n233 = event-data() -> ("CtlRef"=w641:refnum<vi>)  [unwired: 1 in]
        n234 = property class="Bool"(reference=w641) -> ("Label.Text"=w640:string)  [unwired: 1 in, 2 out]
        n235 = call-poly "Enqueue Message.vi"("Message"=w640, "Message Queue"=w639) -> ("error out"=w637:errorcluster, "dup Message Queue"=w638:refnum<queue>)  [unwired: 8 in]
      }
      event "Settings": Value Change {
        n236 = event-data() -> ()  [unwired: 1 in, 1 out]
        n237 = call "HMI Pop Up Alpha KB.vi"("Password Display (F)"=TRUE, "Max Length (70)"=12, "Message In"="Please enter your password") -> ("String Out"=w644:string)  [unwired: 7 in, 1 out]
        n238 = Equal?(x=w644, y=w645) -> (x = y?=w643:bool)
        n239 = case shown="True" w643 {
          tunnel: w651 -> [w653 w658]
          tunnel: [w653 w657] -> w650
          tunnel: [_ w656] -> w649
          tunnel: "Settings Mode Change" -> [_ w654]
          frame False {
            n240 = One Button Dialog(message="Incorrect Password") -> ()  [unwired: 1 in, 1 out]
          }
          frame True {
            n241 = call-poly "Enqueue Message.vi"("Message Data"=w654, "Message"="Settings" ("Message In"), "Message Queue"=w658) -> ("error out"=w656:errorcluster, "dup Message Queue"=w657:refnum<queue>)  [unwired: 7 in]
          }
        }
      }
      event "Settings Mode Change": Value Change {
        n242 = event-data() -> ("NewVal"=w661:T10)  [unwired: 1 in, 5 out]
        n243 = call-poly "Enqueue Message.vi"("error in (no error)"=w660, "Message Data"=w661, "Message"="Settings", "Message Queue"=w664) -> ("error out"=w659:errorcluster, "dup Message Queue"=w663:refnum<queue>)  [unwired: 6 in]
      }
      event "Keyboard 2": Value Change {
        n244 = event-data() -> ()  [unwired: 1 in, 6 out]
        n245 = call <vilib>:"System Exec.vi"("command line"="osk.exe") -> ()  [unwired: 7 in, 4 out]
      }
      event "Clamp", "De-Clamp", "Go Up", "Go Down", "Shipping Position", "Homing": Value Change {
        n246 = event-data() -> ("CtlRef"=w674:refnum<vi>)  [unwired: 1 in]
        n247 = property class="Bool"(reference=w674) -> ("Label.Text"=w670:string)  [unwired: 1 in, 2 out]
        n248 = call-poly "Enqueue Message.vi"("Message Data"=w670, "Message"="Manual Test", "Message Queue"=w673) -> ("error out"=w671:errorcluster, "dup Message Queue"=w672:refnum<queue>)  [unwired: 7 in]
        n249 = for {
          tunnel: w668 -> [w676] mode=indexing
          tunnel: T18."Disabled and Grayed Out" ("Disabled") -> [w675]
          n250 = property class="Bool"(reference=w676, "DisabledEnum"=w675) -> ()  [unwired: 1 in, 2 out]
        }
      }
      event "Home Calib", "Home Settings", "Home Manual": Value Change {
        n251 = event-data() -> ()  [unwired: 1 in, 1 out]
        n252 = call-poly "Enqueue Message.vi"("Message"="Initialize", "Message Queue"=w679) -> ("error out"=w677:errorcluster, "dup Message Queue"=w678:refnum<queue>)  [unwired: 8 in]
      }
      event "Home Maint": Value Change {
        n253 = event-data() -> ()  [unwired: 1 in, 1 out]
        n254 = call-poly "Enqueue Message.vi"("Message"="Exit Maintenance", "Message Queue"=w683) -> ("error out"=w681:errorcluster, "dup Message Queue"=w682:refnum<queue>)  [unwired: 8 in]
      }
      event "Clamp", "Motor Short", "Motor ON", "Motor CW", "Motor CCW", "Load Lift Up Rear", "Load Lift Up Front", "Load Lift Dn Front", "Load Lift Dn Rear", "Loadcell CYL": Value Change {
        n255 = event-data() -> ("CtlRef"=w700:refnum<vi>)  [unwired: 1 in]
        n256 = property class="Bool (strict)"(reference=w700) -> ("Label.Text"=w699:string)  [unwired: 1 in, 2 out]
        n257 = Build Array("Load Lift Up Rear", "Load Lift Up Front", "Load Lift Dn Rear", "Load Lift Dn Front") -> (w690:bool[])
        n258 = Build Array("Loadcell CYL") -> (w686:bool[])
        n259 = Build Array("Clamp") -> (w697:bool[])
        n260 = Build Array("Motor ON", "Motor CW", "Motor CCW", "Motor Short") -> (w693:bool[])
        n261 = case shown="\"Load Lift Dn Front\", \"Load Lift Dn Rear\", \"Load Lift Up Front\", \"Load Lift Up Rear\"" w699 {
          tunnel: w697 -> [w703 _ _ _ _]
          tunnel: w693 -> [_ _ w707 _ _]
          tunnel: w690 -> [_ _ _ w708 _]
          tunnel: w686 -> [_ w704 _ _ _]
          frame "Clamp" {
            n262 = call "FGV - DO.vi"("Digital Outs"=w703, "State"=FGV_DO."Clamping") -> ()  [unwired: 8 in, 2 out]
          }
          frame "Loadcell CYL" {
            n263 = call "FGV - DO.vi"("Digital Outs"=w704, "State"=FGV_DO."Loadcell CYL") -> ()  [unwired: 8 in, 2 out]
          }
          frame "Motor CCW", "Motor CW", "Motor ON", "Motor Short" {
            n264 = call "FGV - DO.vi"("Digital Outs"=w707, "State"=FGV_DO."Contactors") -> ()  [unwired: 8 in, 2 out]
          }
          frame "Load Lift Dn Front", "Load Lift Dn Rear", "Load Lift Up Front", "Load Lift Up Rear" {
            n265 = call "FGV - DO.vi"("Digital Outs"=w708, "State"=FGV_DO."Load CYL") -> ()  [unwired: 8 in, 2 out]
          }
          frame Default {
          }
        }
      }
      event "TareStroke": Value Change {
        n266 = event-data() -> ()  [unwired: 1 in, 5 out]
        n267 = global write "All Inputs.vi" "TareStroke"(TRUE ("TareStroke")) -> ()
      }
      event "TL Red", "TL Orange", "TL Green", "TL Buzzer": Value Change {
        n268 = event-data() -> ()  [unwired: 1 in, 5 out]
        n269 = Build Array("TL Red", "TL Orange", "TL Green", "TL Buzzer") -> (w716:bool[])
        n270 = Boolean Array To Number(Boolean array=w716) -> (number=w717:u32)
        n271 = global write "Towerlight GV.vi" "Maint DO"(w717) -> ()
      }
      event "Save Specs": Value Change {
        n272 = event-data() -> ()  [unwired: 1 in, 1 out]
        n273 = call-poly "Enqueue Message.vi"("Message"="Save Specs", "Message Queue"=w721) -> ("error out"=w719:errorcluster, "dup Message Queue"=w720:refnum<queue>)  [unwired: 8 in]
      }
      event "Home Autocycle": Value Change {
        n274 = event-data() -> ()  [unwired: 1 in, 1 out]
        n275 = Unbundle By Name(w724) -> ("Auto"=w726:refnum<queue>)
        n276 = call-poly "Enqueue Message.vi"("Message"="End Auto Mode", "Message Queue"=w726) -> ("error out"=w723:errorcluster)  [unwired: 8 in, 1 out]
        n277 = call-poly "Enqueue Message.vi"("error in (no error)"=w723, "Message"="Initialize", "Message Queue"=w729) -> ("error out"=w727:errorcluster, "dup Message Queue"=w728:refnum<queue>)  [unwired: 7 in]
      }
      event "Save": Value Change {
        n278 = event-data() -> ()  [unwired: 1 in, 1 out]
        n279 = call-poly "Enqueue Message.vi"("Message"="Update Calibrate", "Message Queue"=w733) -> ("error out"=w731:errorcluster, "dup Message Queue"=w732:refnum<queue>)  [unwired: 8 in]
      }
      event "Print": Value Change {
        n280 = event-data() -> ()  [unwired: 1 in, 1 out]
        n281 = call-poly "Enqueue Message.vi"("Message"="Test Print", "Message Queue"=w737) -> ("error out"=w735:errorcluster, "dup Message Queue"=w736:refnum<queue>)  [unwired: 8 in]
      }
      event "View Log": Value Change {
        n282 = event-data() -> ()  [unwired: 1 in, 1 out]
        n283 = local read "File Path Control"() -> (w739:path)
        n284 = call "View Log.vi"("file path"=w739) -> ()  [unwired: 10 in, 1 out]
      }
      event "Exit": Value Change {
        n285 = event-data() -> ()  [unwired: 1 in, 1 out]
        n286 = call-poly "Enqueue Message.vi"("Priority Message? (F)"=TRUE, "Message"="Exit", "Message Queue"=w745) -> ("error out"=w744:errorcluster, "dup Message Queue"=w743:refnum<queue>)  [unwired: 7 in]
      }
      event User Event {
        # "The Message Handling Loop processed an \"Exit\" message, which fired this event to stop the Event Handling Loop."
        n287 = event-data() -> ()  [unwired: 1 in, 1 out]
      }
    }
    n288 = call "Error Handler - Event Handling Loop.vi"("error in (no error)"=w624, "Message Queue"=w622) -> ("dup error in"=w621:errorcluster)  [unwired: 8 in, 1 out]
  }
  n289 = call "Auto Loop.vi"("error in"=w2, "semaphore"=w28, "Queues in"=w64) -> ("error out"=w65:errorcluster, "semaphore out"=w29:T15)  [unwired: 7 in]
  n290 = call "Towerlight.vi"("error in"=w2, "Notifier in"=w3) -> ("error out"=w66:errorcluster, "Notifier out"=w60:refnum<notifier>)  [unwired: 8 in]
  n291 = for {
    tunnel: w17 -> [w748] mode=indexing
    tunnel: [w748] -> w16 mode=indexing
  }
  "Array" <- w16
  n292 = Unregister For Events(event registration refnum=w71, error in=w69) -> (error out=w72:errorcluster)
  n293 = Merge Errors(w72, w76, w65, w66, w39, w1) -> (w73:errorcluster)
  n294 = flat-sequence {
    tunnel: w73 -> [_]
    tunnel: [w753] -> w70
    tunnel: w67 -> [w752]
    tunnel: w60 -> [w751]
    tunnel: refnum<k21> "1903_Counter" ("task/channels in") -> [w750]
    tunnel: w29 -> [w749]
    frame #0 {
      n295 = call <vilib>:"Release Semaphore Reference.vi"("semaphore"=w749) -> ()  [unwired: 9 in, 2 out]
      n296 = Release Notifier(notifier=w751) -> ()  [unwired: 2 in, 3 out]
      n297 = call "Destroy User Event - Stop.vi"("User Event - Stop"=w752) -> ("error out"=w753:errorcluster)  [unwired: 10 in]
      n298 = call <vilib>:"DAQmx Clear Task.vi"("task in"=w750) -> ()  [unwired: 14 in, 1 out]
    }
  }
  n299 = disable-structure shown="RUN_TIME_ENGINE==True" {
    disable-tunnel: w70 -> [_ _]
    frame condition #0 (active) {
    }
    frame condition #1 {
      # "Call Quit LabVIEW if running as a built application."
      n300 = Quit LabVIEW() -> ()  [unwired: 1 in]
    }
  }
